vi "COD主界面（列队使用）.vi"() -> (8 "多列列表框":i32(listbox))   [LabVIEW 2016, in "斯坦道CODMn.lvlib"]
uses:
  <vilib>/Analysis/6fits.llb/Curve Fitting Criteria.ctl
  <vilib>/Utility/miscctls.llb/LVPointTypeDef.ctl
  <vilib>/Plasmionique/MB Master/MB_Master_Serial/MB_Master_Serial.lvclass
  F:/Program Files/National Instruments/LabVIEW 2016/vi.lib/Plasmionique/MB Master/MB_Master/MB_Master.lvclass
  <vilib>/Utility/config.llb/Read Key (Double).vi
  <vilib>/Utility/config.llb/Read Key (I32).vi
  <vilib>/Utility/config.llb/Read Key (Boolean).vi
  <vilib>/Utility/config.llb/Write Key (I32).vi
  <vilib>/Utility/config.llb/Write Key (Double).vi
  <vilib>/Utility/config.llb/Write Key (Boolean).vi
  <vilib>/Plasmionique/MB Master/MB Master.lvlib
  <vilib>/ptbypt/NI_PtbyPt.lvlib
  PLC/PLC.lvlib
  <vilib>/Utility/config.llb/NI_LVConfig.lvlib
  <vilib>/Analysis/NI_AALPro.lvlib
panel:
  in  "方程参数写入":bool
  in  "读取方程系数":T1
  out "高量程拟合方程":string
  out "低量程拟合方程":string
  out "测量模式数字":i32
  out "零点核查标记":bool
  out "排液故障":bool
  out "进水样超量程":bool
  out "标样核查标记":bool
  out "平行样测量":bool
  out "加标回收测量":bool
  out "质控样测量":bool
  out "待机":bool
  out "校标错误":bool
  out "校零错误":bool
  out "测量错误":bool
  out "草酸钠报警":bool
  out "高锰酸钾报警":bool
  out "加热故障":bool
  out "温控器故障":bool
  out "ORP故障":bool
  out "排液标记":bool
  out "故障标记":bool
  out "校标标记":bool
  out "校零标记":bool
  out "通讯状态":bool
  out "水样测量":bool
  out "读取KB值":bool
  in  "读取":bool
  out "b 2":dbl
  out "K 2":dbl
  out "b":dbl
  out "K":dbl
  out "当前选用的校准":i32
  in  "启用3":bool
  in  "启用2":bool
  in  "启用1":bool
  in  "启用6":bool
  in  "启用5":bool
  in  "校准6":bool
  in  "校准5":bool
  in  "校准4":bool
  in  "启用4":bool
  in  "泵滴定数6":dbl
  in  "泵滴定数5":dbl
  in  "泵滴定数4":dbl
  in  "浓度6":dbl
  in  "浓度5":dbl
  in  "浓度4":dbl
  in  "校准3":bool
  in  "校准2":bool
  in  "校准1":bool
  in  "泵滴定数3":dbl
  in  "泵滴定数2":dbl
  in  "泵滴定数1":dbl
  in  "浓度3":dbl
  in  "浓度2":dbl
  in  "浓度1":dbl
  in  "返回":bool
  in  "校准配置":bool
  in  "修正系数 2":dbl
  in  "浓度 2":dbl
  in  "温度":dbl
  in  "保存":bool
  in  "恒温时间":dbl
  in  "基本量程":enum16{"10mL", "20mL"}(ring)
  in  "水样":dbl
  in  "蒸馏水":dbl
  in  "标液":dbl
  in  "质控样":dbl
  in  "加标回收":dbl
  in  "草酸钠":dbl
  in  "高锰酸钾":dbl
  in  "硫酸":dbl
  in  "关闭":bool
  in  "零点泵计量数 2":dbl
  in  "标度泵计量数 2":dbl
  out "标度滴定值":dbl
  out "零点滴定值":dbl
  out "测量数据区":T2 {"单位" items=["ug/L", "mg/L", "ppm", "mg/m3", "cm", "ppb", "ug/m3", "%", "nmol/mol", "umol/mol", "MPN/L", "MPN/100ml", "ng/m3", "NTU", "无量纲", "ms/cm", "us/cm", "℃", "mV", "万个/L"]}
  out "启动选择 3":u16(ring) items=["水样测试", "标样核查", "零点核查", "加标回收", "平行样", "校零", "校标", ""]
  out "仪器时间":timestamp
  out "秒":u16
  out "分":u16
  out "COD浓度（mg/L)":dbl format="%.2g"
  out "进样管":dbl
  out "高锰酸钾":dbl
  out "草酸钠":dbl
  out "硫酸":dbl
  out "ORP显示":dbl
  out "温度":dbl
  out "加热":bool
  out "搅拌":bool
  out "进硫酸":bool
  out "进加标回收样":bool
  out "进质控样":bool
  out "进标液":bool
  out "进蒸馏水":bool
  out "进水样":bool
  out "进草酸钠":bool
  out "进高锰酸钾":bool
  in  "定时启动":bool
  in  "启动":bool
  in  "故障清除":bool
  in  "参数配置":bool
  in  "停止":bool
  in  "单步启动":bool
  out "设置值":dbl
  out "系统时间":timestamp
  in  "时间校准":bool
  in  "枚举":enum16{"读取数据", "写入数据", "读取写入DATABASE", "读取参数"}(ring)
  in  "data in":T3
  out "数值":i32
  out "报警簇":T4
  out "读取参数":u16[](array[numeric])
  out "循环次数":i32
  out "DATABASE":u16[](array[numeric])
  out "Registers":u16[](array[numeric])
  in  "Slave ID":u8=1
  in  "Serial Config":T5={"baud rate (bps)"=115200, "stop bits"=10, "parity"=0, "flow control"=0, "timeout"=1000, "retries"=1} {"stop bits" items=["1.0"=10, "1.5"=15, "2.0"=20]; "flow control" items=["None", "XON/XOFF", "RTS/CTS", "XON/XOFF & RTS/CTS", "DTR/DSR", "XON/XOFF & DTR/DSR"]; "parity" items=["None", "Odd", "Even", "Mark", "Space"]}
  out "table 输入":string
  out "columns":string[](array[string])
  out "data":T6
  in  "温度 2":dbl
  in  "浓度":dbl
  in  "修正系数":dbl
  in  "标样浓度 2":dbl
  out "模式（受控）":u16
  in  "VISA resource name":refnum<visa-resource-name>="COM3" caption="VISA资源名称"
  # "测量时间："
  # "水样~加标回收"
  # "mV"
  # "℃"
  # "注：遇到加热故障和排液故障时仪器不能正常启动，\n必须排查故障并点击报警清除按钮方可运行。"
  # "mg/L"
  # "基本参数设置"
  # "泵计量参数设置"
  # "校零校标结果"
  # "加热恒温温度（℃）："
  # "水样："
  # "高锰酸钾："
  # "校零结果："
  # "校零滴定值："
  # "恒温时间（分钟）："
  # "蒸馏水："
  # "草酸钠："
  # "校标结果："
  # "标度滴定值："
  # "零点泵计量值："
  # "标准液浓度（mg/L）："
  # "标液："
  # "硫酸："
  # "标样浓度："
  # "标度泵计量值："
  # "修正系数："
  # "质控样："
  # "加标回收样："
  # "基本量程（20mL可选）："
  # "低量程校准"
  # "高量程校准"
  # "泵滴定数"
  # "是否启用"
  # "泵滴定数"
  # "是否启用"
  # "浓度"
  # "浓度"
  # "将方程写入"
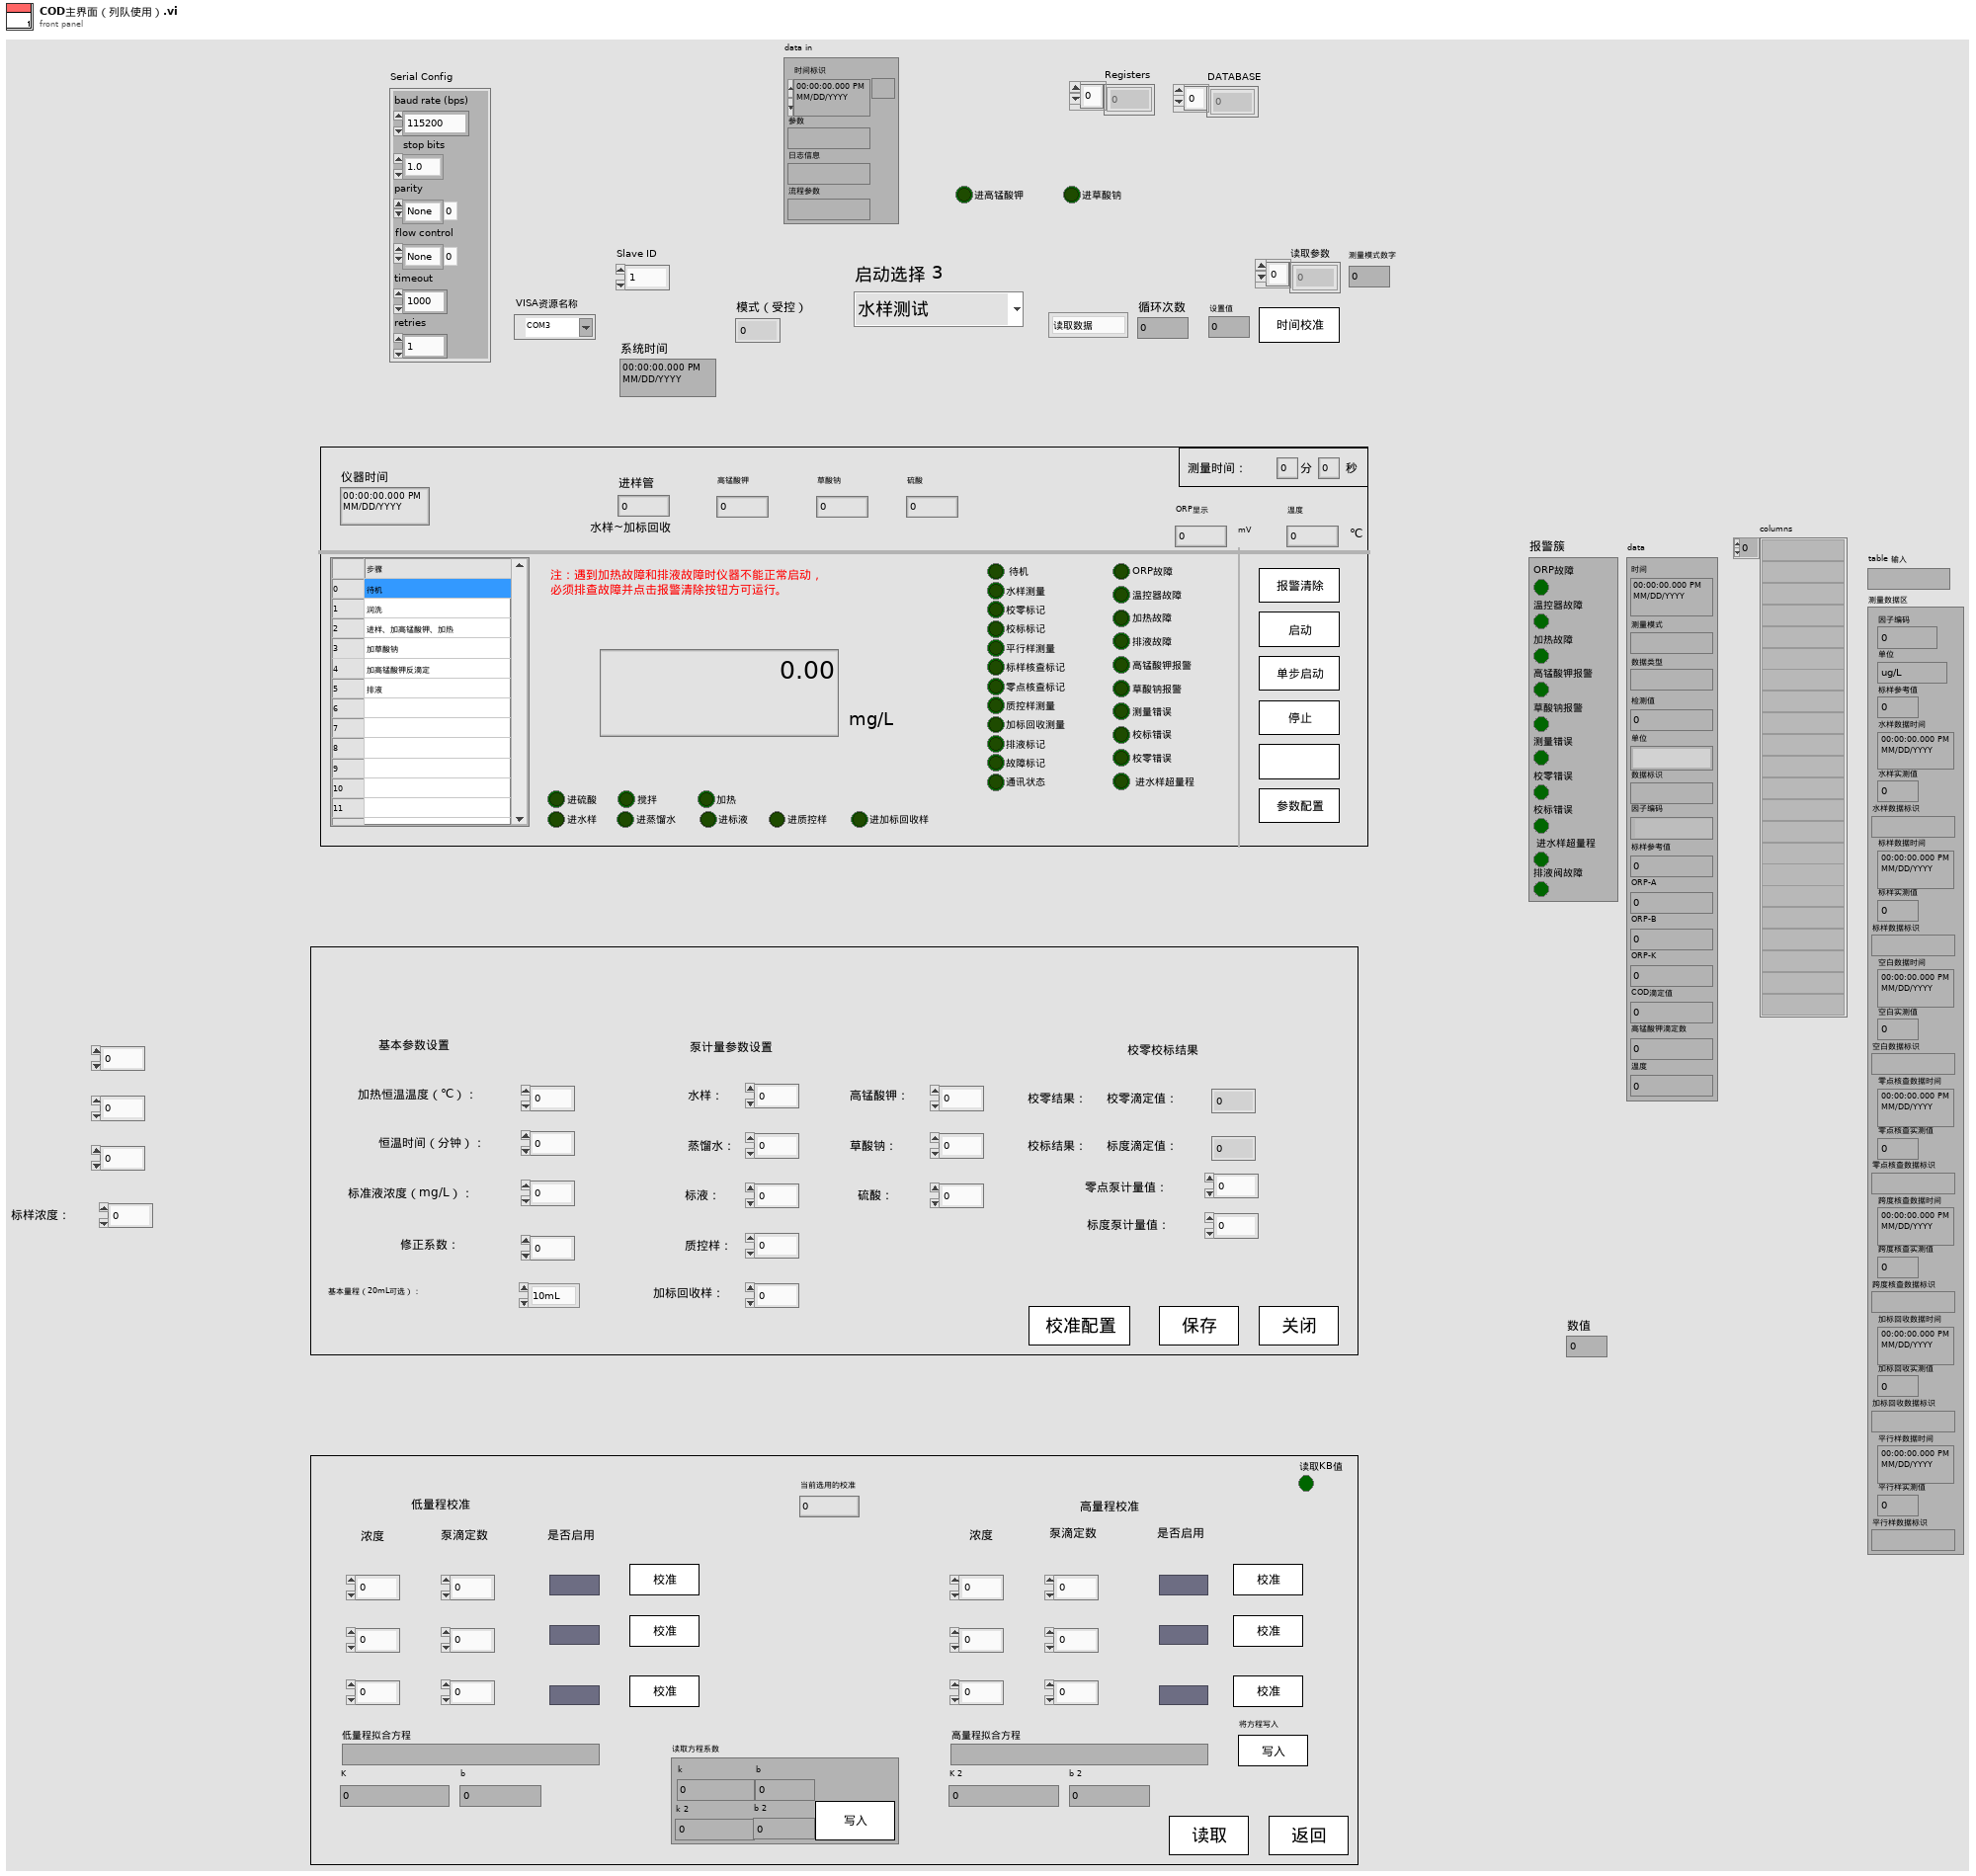
[diagram p1: front panel]
types:
  T1 = cluster{"k":dbl, "b":dbl, "k 2":dbl, "b 2":dbl, "写入":bool}
  T2 = cluster{"因子编码":u32, "单位":u16, "标样参考值":sgl, "水样数据时间":timestamp, "水样实测值":sgl, "水样数据标识":string, "标样数据时间":timestamp, "标样实测值":sgl, "标样数据标识":string, "空白数据时间":timestamp, "空白实测值":sgl, "空白数据标识":string, "零点核查数据时间":timestamp, "零点核查实测值":sgl, "零点核查数据标识":string, "跨度核查数据时间":timestamp, "跨度核查实测值":sgl, "跨度核查数据标识":string, "加标回收数据时间":timestamp, "加标回收实测值":sgl, "加标回收数据标识":string, "平行样数据时间":timestamp, "平行样实测值":sgl, "平行样数据标识":string}
  T3 = cluster{"时间标识":timestamp, "参数":string, "日志信息":string, "流程参数":string}
  T4 = cluster{"ORP故障":bool, "温控器故障":bool, "加热故障":bool, "高锰酸钾报警":bool, "草酸钠报警":bool, "测量错误":bool, "校零错误":bool, "校标错误":bool, " 进水样超量程":bool, "排液阀故障":bool}
  T5 = cluster{"baud rate (bps)":u32, "stop bits":u16, "parity":u16, "flow control":u16, "timeout":u32, "retries":i32}
  T6 = cluster{"时间":timestamp, "测量模式":string, "数据类型":string, "检测值":sgl, "单位":string, "数据标识":string, "因子编码":string, "标样参考值":sgl, "ORP-A":sgl, "ORP-B":sgl, "ORP-K":sgl, "COD滴定值":sgl, "高锰酸钾滴定数":sgl, "温度":sgl}
  T7 = cluster{"starting address":u16, "number of holding registers":u16}
  T8 = typedef "LVPointTypeDef.ctl" = cluster{"Horizontal":i16, "Vertical":i16}
  T9 = cluster{"测量模式":enum16{"水样测量", "标样核查", "零点核查", "加标回收", "平行样", "校零", "校标"}}
  T10 = typedef "NI_LVConfig.lvlib/Config Data RefNum.ctl" = refnum<k1>
  T11 = cluster{"时间标识":timestamp, "设备":string, "日志信息":string}
  T12 = typedef "NI_AALPro.lvlib/Curve Fitting Criteria.ctl" = u16
  T13 = cluster{"时间标识":timestamp, "设备":string, "日志信息":string, "流程参数":string}
  T14 = cluster{"数组 2[0]":sgl, "数组 2[1]":sgl, "数组 2[2]":sgl, "数组 2[3]":sgl}
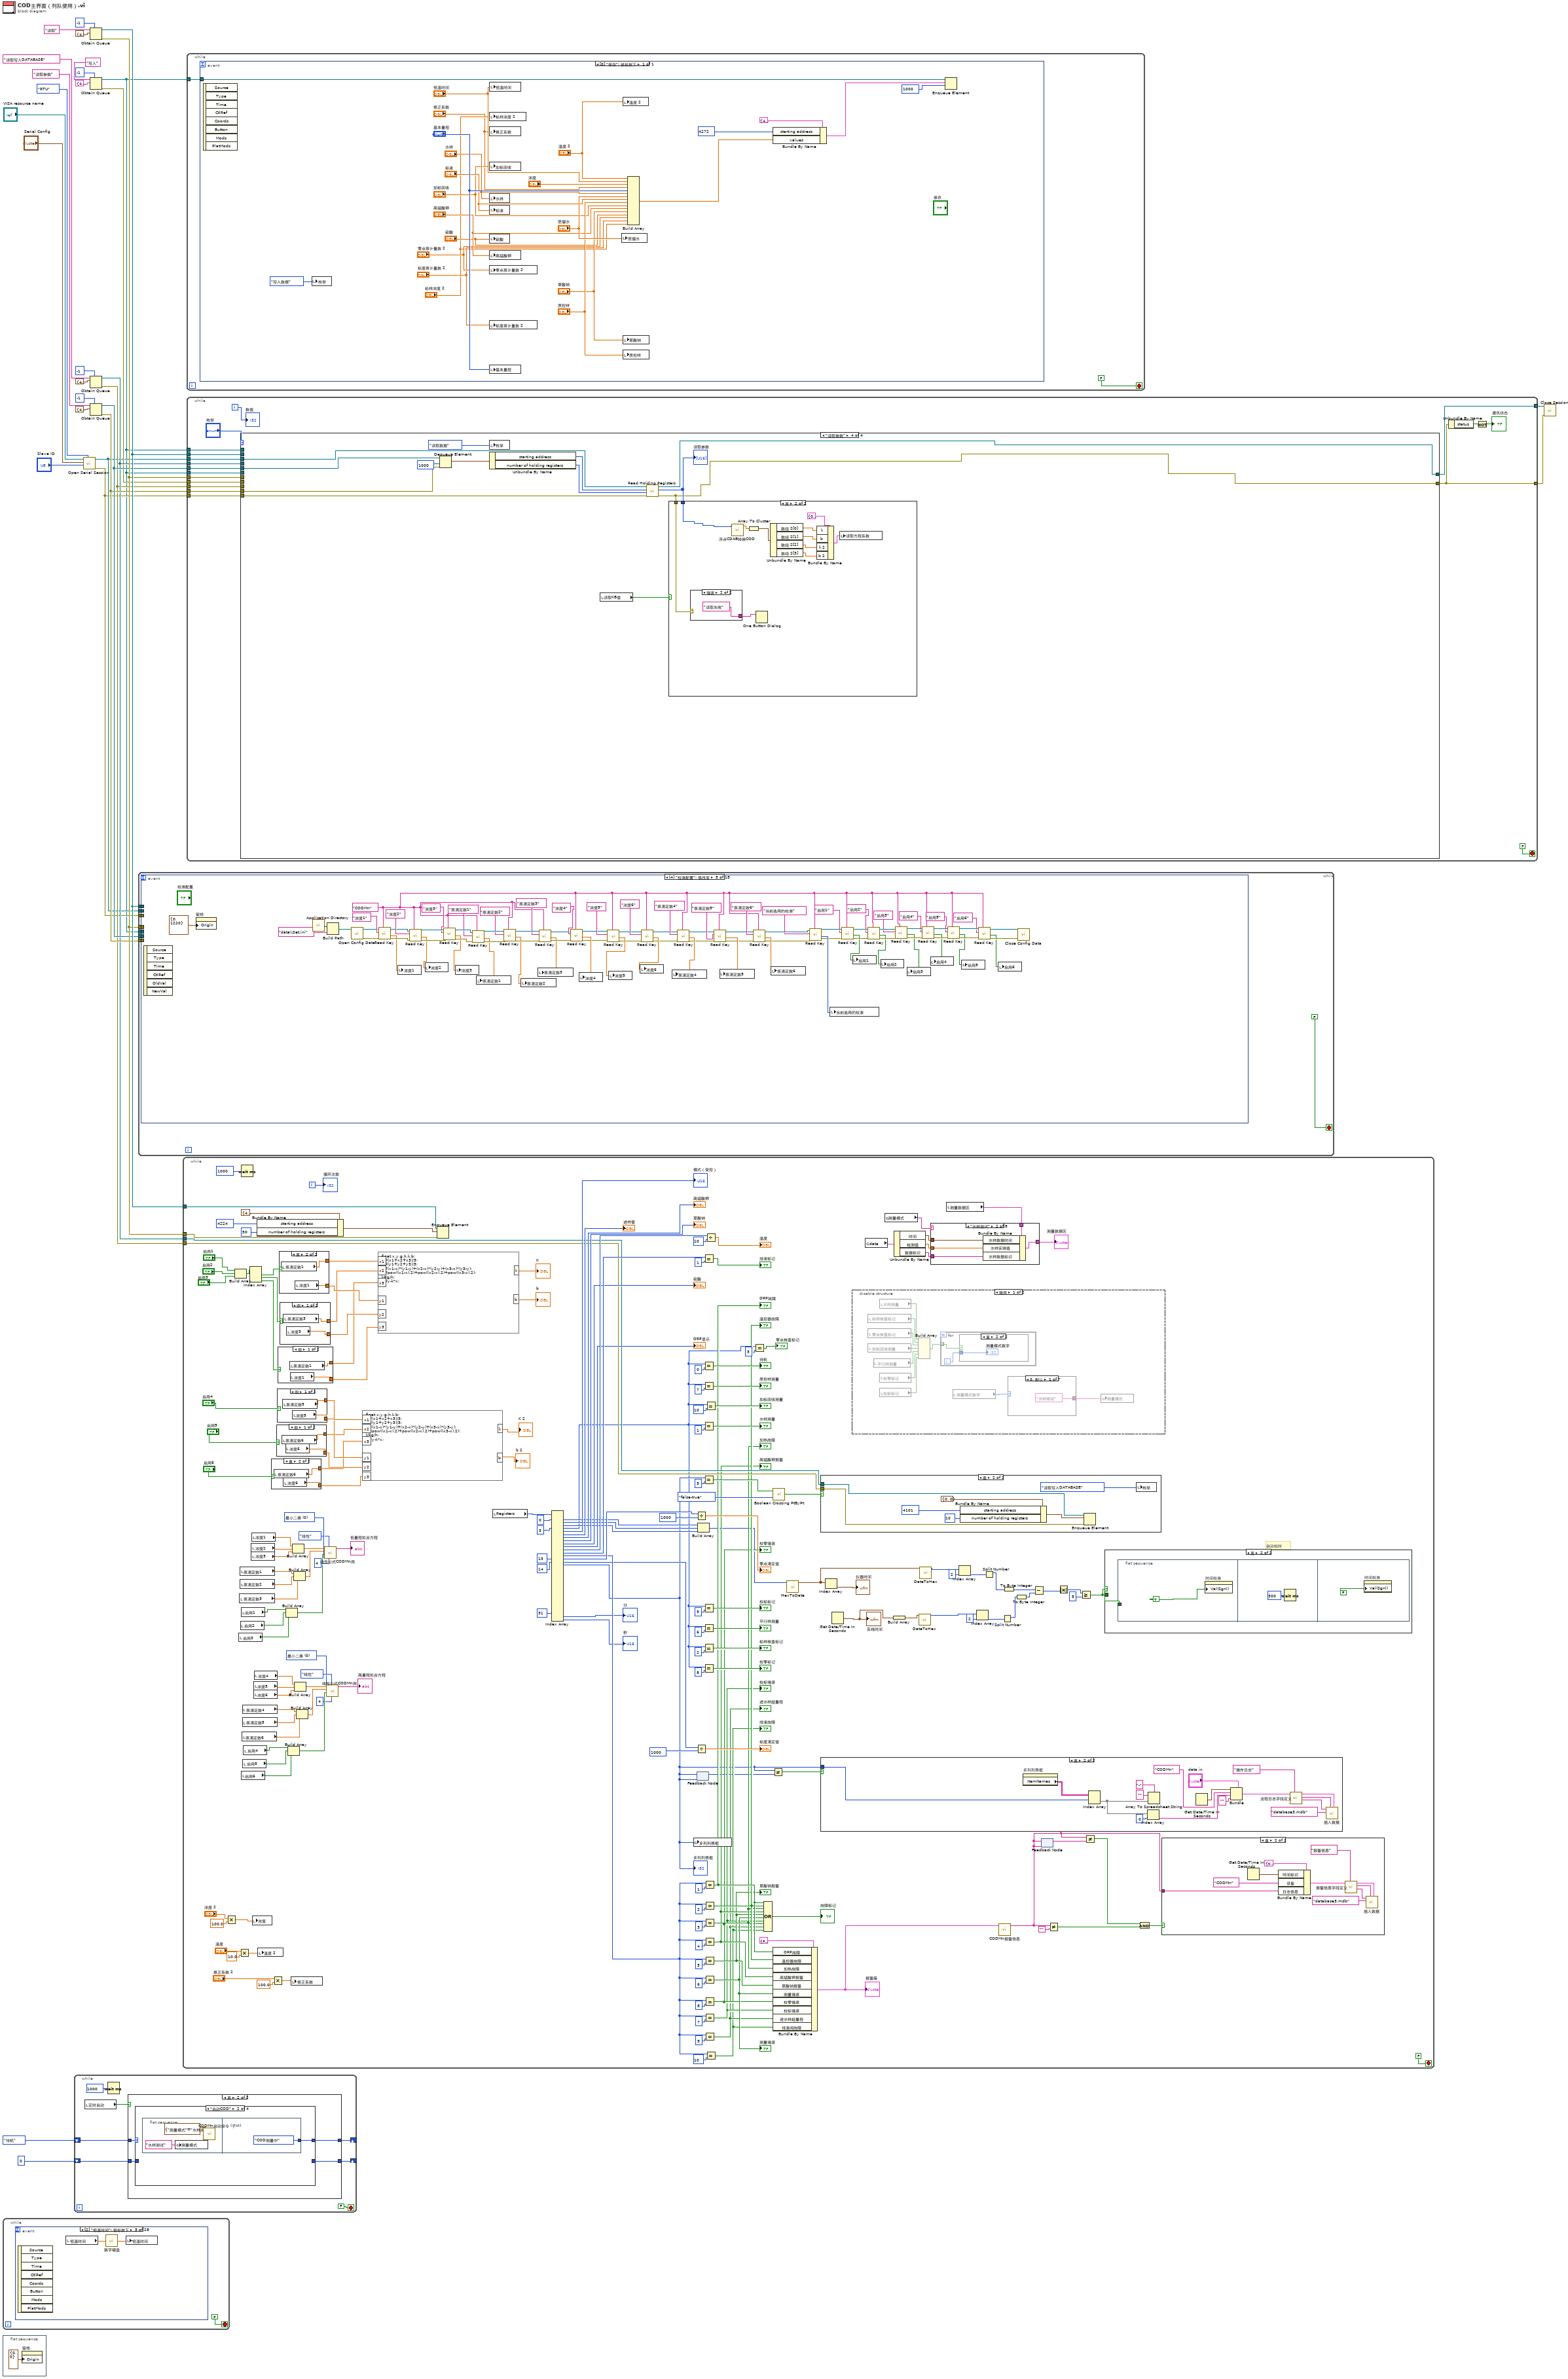
[diagram p0: block diagram]
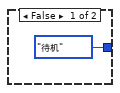
[diagram p2: hidden frame]
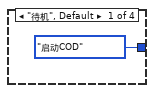
[diagram p3: hidden frame]
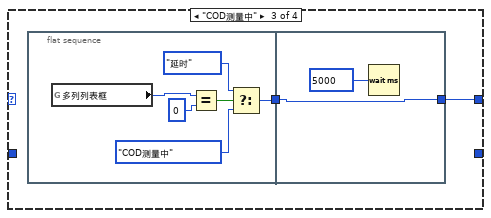
[diagram p4: hidden frame]
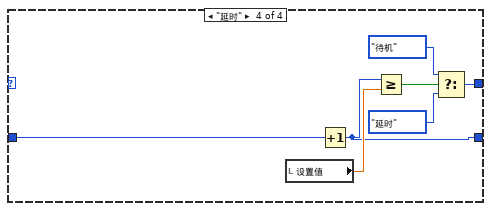
[diagram p5: hidden frame]
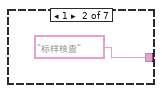
[diagram p6: hidden frame]
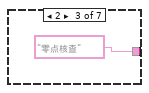
[diagram p7: hidden frame]
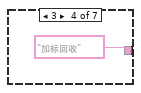
[diagram p8: hidden frame]
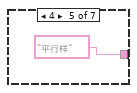
[diagram p9: hidden frame]
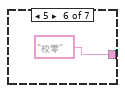
[diagram p10: hidden frame]
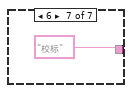
[diagram p11: hidden frame]
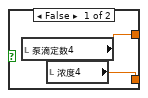
[diagram p14: hidden frame]
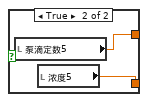
[diagram p15: hidden frame]
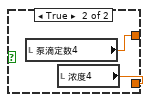
[diagram p16: hidden frame]
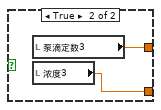
[diagram p17: hidden frame]
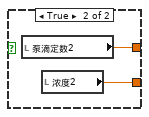
[diagram p18: hidden frame]
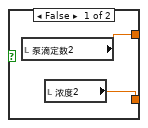
[diagram p19: hidden frame]
diagram:
  n1 = while {
    stop <- FALSE stop-if-true
    n2 = event shown="[2] \"恒温时间\": 鼠标按下" {
      selector: _ -> [_ _ _ _ _ _ _ _ _ _ _ _ _ _ _ _ _ _ _ _ _ _ _ _ _ _ _ _]
      dyn-events: _ -> [_ _ _ _ _ _ _ _ _ _ _ _ _ _ _ _ _ _ _ _ _ _ _ _ _ _ _ _]
      timeout: _ -> [_ _ _ _ _ _ _ _ _ _ _ _ _ _ _ _ _ _ _ _ _ _ _ _ _ _ _ _]
      event Timeout {
        n3 = event-data() -> ()  [unwired: 1 in, 3 out]
      }
      event "温度": Mouse Down {
        n4 = event-data() -> ()  [unwired: 1 in, 8 out]
        n5 = local read "温度"() -> (w33:dbl)
        n6 = call "数字键盘.vi"("OldNumber"=w33) -> ("NewNumber"=w32:sgl)
        n7 = local write "温度"(w32) -> ()
      }
      event "恒温时间": Mouse Down {
        n8 = event-data() -> ()  [unwired: 1 in, 8 out]
        n9 = local read "恒温时间"() -> (w34:dbl)
        n10 = call "数字键盘.vi"("OldNumber"=w34) -> ("NewNumber"=w35:sgl)
        n11 = local write "恒温时间"(w35) -> ()
      }
      event "浓度 2": Mouse Down {
        n12 = event-data() -> ()  [unwired: 1 in, 8 out]
        n13 = local read "浓度 2"() -> (w37:dbl)
        n14 = call "数字键盘.vi"("OldNumber"=w37) -> ("NewNumber"=w36:sgl)
        n15 = local write "浓度 2"(w36) -> ()
      }
      event "修正系数 2": Mouse Down {
        n16 = event-data() -> ()  [unwired: 1 in, 8 out]
        n17 = local read "修正系数 2"() -> (w38:dbl)
        n18 = call "数字键盘.vi"("OldNumber"=w38) -> ("NewNumber"=w39:sgl)
        n19 = local write "修正系数 2"(w39) -> ()
      }
      event "水样": Mouse Down {
        n20 = event-data() -> ()  [unwired: 1 in, 8 out]
        n21 = local read "水样"() -> (w40:dbl)
        n22 = call "数字键盘.vi"("OldNumber"=w40) -> ("NewNumber"=w41:sgl)
        n23 = local write "水样"(w41) -> ()
      }
      event "蒸馏水": Mouse Down {
        n24 = event-data() -> ()  [unwired: 1 in, 8 out]
        n25 = local read "蒸馏水"() -> (w42:dbl)
        n26 = call "数字键盘.vi"("OldNumber"=w42) -> ("NewNumber"=w43:sgl)
        n27 = local write "蒸馏水"(w43) -> ()
      }
      event "标液": Mouse Down {
        n28 = event-data() -> ()  [unwired: 1 in, 8 out]
        n29 = local read "标液"() -> (w44:dbl)
        n30 = call "数字键盘.vi"("OldNumber"=w44) -> ("NewNumber"=w45:sgl)
        n31 = local write "标液"(w45) -> ()
      }
      event "质控样": Mouse Down {
        n32 = event-data() -> ()  [unwired: 1 in, 8 out]
        n33 = local read "质控样"() -> (w46:dbl)
        n34 = call "数字键盘.vi"("OldNumber"=w46) -> ("NewNumber"=w47:sgl)
        n35 = local write "质控样"(w47) -> ()
      }
      event "加标回收": Mouse Down {
        n36 = event-data() -> ()  [unwired: 1 in, 8 out]
        n37 = local read "加标回收"() -> (w48:dbl)
        n38 = call "数字键盘.vi"("OldNumber"=w48) -> ("NewNumber"=w49:sgl)
        n39 = local write "加标回收"(w49) -> ()
      }
      event "草酸钠": Mouse Down {
        n40 = event-data() -> ()  [unwired: 1 in, 8 out]
        n41 = local read "草酸钠"() -> (w50:dbl)
        n42 = call "数字键盘.vi"("OldNumber"=w50) -> ("NewNumber"=w51:sgl)
        n43 = local write "草酸钠"(w51) -> ()
      }
      event "高锰酸钾": Mouse Down {
        n44 = event-data() -> ()  [unwired: 1 in, 8 out]
        n45 = local read "高锰酸钾"() -> (w52:dbl)
        n46 = call "数字键盘.vi"("OldNumber"=w52) -> ("NewNumber"=w53:sgl)
        n47 = local write "高锰酸钾"(w53) -> ()
      }
      event "硫酸": Mouse Down {
        n48 = event-data() -> ()  [unwired: 1 in, 8 out]
        n49 = local read "硫酸"() -> (w54:dbl)
        n50 = call "数字键盘.vi"("OldNumber"=w54) -> ("NewNumber"=w55:sgl)
        n51 = local write "硫酸"(w55) -> ()
      }
      event "零点泵计量数 2": Mouse Down {
        n52 = event-data() -> ()  [unwired: 1 in, 8 out]
        n53 = local read "零点泵计量数 2"() -> (w56:dbl)
        n54 = call "数字键盘.vi"("OldNumber"=w56) -> ("NewNumber"=w57:sgl)
        n55 = local write "零点泵计量数 2"(w57) -> ()
      }
      event "标度泵计量数 2": Mouse Down {
        n56 = event-data() -> ()  [unwired: 1 in, 8 out]
        n57 = local read "标度泵计量数 2"() -> (w58:dbl)
        n58 = call "数字键盘.vi"("OldNumber"=w58) -> ("NewNumber"=w59:sgl)
        n59 = local write "标度泵计量数 2"(w59) -> ()
      }
      event "标样浓度 2": Mouse Down {
        n60 = event-data() -> ()  [unwired: 1 in, 8 out]
        n61 = local read "标样浓度 2"() -> (w60:dbl)
        n62 = call "数字键盘.vi"("OldNumber"=w60) -> ("NewNumber"=w61:sgl)
        n63 = local write "标样浓度 2"(w61) -> ()
      }
      event "浓度1": Mouse Down {
        n64 = event-data() -> ()  [unwired: 1 in, 8 out]
        n65 = local read "浓度1"() -> (w63:dbl)
        n66 = call "数字键盘.vi"("OldNumber"=w63) -> ("NewNumber"=w62:sgl)
        n67 = property on="浓度1" class="DigNum (严格)"("Val(Sgnl)"=w62) -> ()  [unwired: 2 in, 2 out]
      }
      event "浓度2": Mouse Down {
        n68 = event-data() -> ()  [unwired: 1 in, 8 out]
        n69 = local read "浓度2"() -> (w65:dbl)
        n70 = call "数字键盘.vi"("OldNumber"=w65) -> ("NewNumber"=w64:sgl)
        n71 = property on="浓度2" class="DigNum (严格)"("Val(Sgnl)"=w64) -> ()  [unwired: 2 in, 2 out]
      }
      event "浓度3": Mouse Down {
        n72 = event-data() -> ()  [unwired: 1 in, 8 out]
        n73 = local read "浓度3"() -> (w67:dbl)
        n74 = call "数字键盘.vi"("OldNumber"=w67) -> ("NewNumber"=w66:sgl)
        n75 = property on="浓度3" class="DigNum (严格)"("Val(Sgnl)"=w66) -> ()  [unwired: 2 in, 2 out]
      }
      event "泵滴定数1": Mouse Down {
        n76 = event-data() -> ()  [unwired: 1 in, 8 out]
        n77 = local read "泵滴定数1"() -> (w69:dbl)
        n78 = call "数字键盘.vi"("OldNumber"=w69) -> ("NewNumber"=w68:sgl)
        n79 = property on="泵滴定数1" class="DigNum (严格)"("Val(Sgnl)"=w68) -> ()  [unwired: 2 in, 2 out]
      }
      event "泵滴定数2": Mouse Down {
        n80 = event-data() -> ()  [unwired: 1 in, 8 out]
        n81 = local read "泵滴定数2"() -> (w71:dbl)
        n82 = call "数字键盘.vi"("OldNumber"=w71) -> ("NewNumber"=w70:sgl)
        n83 = property on="泵滴定数2" class="DigNum (严格)"("Val(Sgnl)"=w70) -> ()  [unwired: 2 in, 2 out]
      }
      event "泵滴定数3": Mouse Down {
        n84 = event-data() -> ()  [unwired: 1 in, 8 out]
        n85 = local read "泵滴定数3"() -> (w73:dbl)
        n86 = call "数字键盘.vi"("OldNumber"=w73) -> ("NewNumber"=w72:sgl)
        n87 = property on="泵滴定数3" class="DigNum (严格)"("Val(Sgnl)"=w72) -> ()  [unwired: 2 in, 2 out]
      }
      event "浓度4": Mouse Down {
        n88 = event-data() -> ()  [unwired: 1 in, 8 out]
        n89 = local read "浓度4"() -> (w75:dbl)
        n90 = call "数字键盘.vi"("OldNumber"=w75) -> ("NewNumber"=w74:sgl)
        n91 = property on="浓度4" class="DigNum (严格)"("Val(Sgnl)"=w74) -> ()  [unwired: 2 in, 2 out]
      }
      event "浓度5": Mouse Down {
        n92 = event-data() -> ()  [unwired: 1 in, 8 out]
        n93 = local read "浓度5"() -> (w77:dbl)
        n94 = call "数字键盘.vi"("OldNumber"=w77) -> ("NewNumber"=w76:sgl)
        n95 = property on="浓度5" class="DigNum (严格)"("Val(Sgnl)"=w76) -> ()  [unwired: 2 in, 2 out]
      }
      event "浓度6": Mouse Down {
        n96 = event-data() -> ()  [unwired: 1 in, 8 out]
        n97 = local read "浓度6"() -> (w79:dbl)
        n98 = call "数字键盘.vi"("OldNumber"=w79) -> ("NewNumber"=w78:sgl)
        n99 = property on="浓度6" class="DigNum (严格)"("Val(Sgnl)"=w78) -> ()  [unwired: 2 in, 2 out]
      }
      event "泵滴定数4": Mouse Down {
        n100 = event-data() -> ()  [unwired: 1 in, 8 out]
        n101 = local read "泵滴定数4"() -> (w81:dbl)
        n102 = call "数字键盘.vi"("OldNumber"=w81) -> ("NewNumber"=w80:sgl)
        n103 = property on="泵滴定数4" class="DigNum (严格)"("Val(Sgnl)"=w80) -> ()  [unwired: 2 in, 2 out]
      }
      event "泵滴定数5": Mouse Down {
        n104 = event-data() -> ()  [unwired: 1 in, 8 out]
        n105 = local read "泵滴定数5"() -> (w83:dbl)
        n106 = call "数字键盘.vi"("OldNumber"=w83) -> ("NewNumber"=w82:sgl)
        n107 = property on="泵滴定数5" class="DigNum (严格)"("Val(Sgnl)"=w82) -> ()  [unwired: 2 in, 2 out]
      }
      event "泵滴定数6": Mouse Down {
        n108 = event-data() -> ()  [unwired: 1 in, 8 out]
        n109 = local read "泵滴定数6"() -> (w85:dbl)
        n110 = call "数字键盘.vi"("OldNumber"=w85) -> ("NewNumber"=w84:sgl)
        n111 = property on="泵滴定数6" class="DigNum (严格)"("Val(Sgnl)"=w84) -> ()  [unwired: 2 in, 2 out]
      }
    }
  }
  n112 = flat-sequence {
    frame #0 {
      n113 = property on="窗格" class="Pane"("Origin"=T8 {"Horizontal"=0, "Vertical"=0} ("原点")) -> ()  [unwired: 2 in, 2 out]
    }
  }
  n114 = while {
    shift-right: [w88] -> _
    shift-left: enum16{"待机", "启动COD", "COD测量中", "延时"}."待机" -> [w90]
    shift-right: [w87] -> _
    shift-left: 0 -> [w89]
    stop <- FALSE stop-if-true
    n115 = local read "定时启动"() -> (w92:bool)
    n116 = Wait (ms)(milliseconds to wait=u32 1000 ("等待时间（毫秒）")) -> ()  [unwired: 1 out]
    n117 = case shown="真" w92 {
      tunnel: w90 -> [_ w98]
      tunnel: w89 -> [_ w97]
      tunnel: [enum16{"待机", "启动COD", "COD测量中", "延时"}."待机" w96] -> w88
      tunnel: [_ w95] -> w87
      frame False {
      }
      frame True {
        n118 = case shown="\"启动COD\"" w98 {
          tunnel: w97 -> [_ _ _ w120]
          tunnel: [enum16{"待机", "启动COD", "COD测量中", "延时"}."启动COD" w100 w105 w114] -> w96
          tunnel: [_ _ _ w117] -> w95
          frame "待机", Default {
          }
          frame "启动COD" {
            n119 = flat-sequence {
              tunnel: [enum16{"待机", "启动COD", "COD测量中", "延时"}."COD测量中"] -> w100
              frame #0 {
                n120 = global write "COD测量模式全局.vi" "测量模式"("水样测试" ("测量模式")) -> ()
                n121 = call "CODMn启动命令 (子VI).vi"("启动测量模式"=T9 {"测量模式"=enum."水样测量"}) -> ()  [unwired: 11 in]
              }
              frame #1 {
              }
            }
          }
          frame "COD测量中" {
            n122 = flat-sequence {
              tunnel: [w106] -> w104
              tunnel: [w113] -> w105
              tunnel: w104 -> [w113]
              frame #0 {
                n123 = global read "运行时序全局变量.vi" "多列列表框"() -> (w111:i32)
                n124 = Equal?(x=w111, y=0) -> (x = y?=w109:bool)
                n125 = Select(t=enum16{"待机", "启动COD", "COD测量中", "延时"}."延时", s=w109, f=enum16{"待机", "启动COD", "COD测量中", "延时"}."COD测量中") -> (s? t:f=w106:enum16{"待机", "启动COD", "COD测量中", "延时"})
              }
              frame #1 {
                n126 = Wait (ms)(milliseconds to wait=u32 5000 ("等待时间（毫秒）")) -> ()  [unwired: 1 out]
              }
            }
          }
          frame "延时" {
            n127 = local read "设置值"() -> (w119:dbl)
            n128 = Increment(x=w120) -> (x+1=w117:i32)
            n129 = Greater Or Equal?(x=w117, y=w119) -> (x >= y?=w118:bool)
            n130 = Select(t=enum16{"待机", "启动COD", "COD测量中", "延时"}."待机", s=w118, f=enum16{"待机", "启动COD", "COD测量中", "延时"}."延时") -> (s? t:f=w114:enum16{"待机", "启动COD", "COD测量中", "延时"})
          }
        }
      }
    }
  }
  n131 = call <vilib>:"Open Serial Session.vi"("Mode (RTU)"=enum16{"RTU", "ASCII"}."RTU", "Slave ID"="Slave ID", "Serial Config"="Serial Config", "VISA Resource"="VISA resource name") -> ("Error out"=w4:errorcluster, "MB_Serial session"=w5:refnum<class "MB_Master_Serial.lvclass">)  [unwired: 6 in]
  n132 = Obtain Queue(max queue size (-1, unlimited)=-1 ("队列最大值（-1，无限）"), name (unnamed)="读取" ("名称（未命名）"), element data type=T7 {"starting address"=4224, "number of holding registers"=16}) -> (queue out=w20:refnum<queue>, error out=w19:errorcluster)  [unwired: 2 in, 1 out]
  n133 = Obtain Queue(max queue size (-1, unlimited)=-1 ("队列最大值（-1，无限）"), name (unnamed)="写入" ("名称（未命名）"), element data type=cluster{"starting address":u16, "values":u16[]} {"starting address"=4272, "values"=[]}) -> (queue out=w1:refnum<queue>, error out=w6:errorcluster)  [unwired: 2 in, 1 out]
  n134 = Obtain Queue(max queue size (-1, unlimited)=-1 ("队列最大值（-1，无限）"), name (unnamed)="读取写入DATABASE" ("名称（未命名）"), element data type=T7 {"starting address"=4224, "number of holding registers"=16}) -> (queue out=w8:refnum<queue>, error out=w7:errorcluster)  [unwired: 2 in, 1 out]
  n135 = Obtain Queue(max queue size (-1, unlimited)=-1 ("队列最大值（-1，无限）"), name (unnamed)="读取参数" ("名称（未命名）"), element data type=T7 {"starting address"=4224, "number of holding registers"=16}) -> (queue out=w13:refnum<queue>, error out=w12:errorcluster)  [unwired: 2 in, 1 out]
  n136 = while {
    tunnel: w20 -> [w128]
    tunnel: w19 -> [w127]
    tunnel: w1 -> [w126]
    tunnel: w13 -> [w125]
    tunnel: w12 -> [w124]
    tunnel: w5 -> [w122]
    tunnel: w4 -> [w121]
    stop <- FALSE stop-if-true
    n137 = event shown="[4] \"校准配置\": 值改变" {
      selector: _ -> [_ _ _ _ _ _ _ _ _ _ _ _ _ _ _]
      dyn-events: _ -> [_ _ _ _ _ _ _ _ _ _ _ _ _ _ _]
      timeout: _ -> [_ _ _ _ _ _ _ _ _ _ _ _ _ _ _]
      tunnel: w128 -> [_ _ _ _ _ _ _ _ _ _ _ _ _ _ _]
      tunnel: w127 -> [_ _ _ _ _ _ _ _ _ _ _ _ _ _ _]
      tunnel: w126 -> [w135 w163 w194 _ _ _ _ w297 w311 _ w319 _ _ w479 w496]
      tunnel: w125 -> [_ _ _ w201 _ _ _ _ _ _ _ _ w471 _ _]
      tunnel: w124 -> [_ _ _ w200 _ _ _ _ _ _ _ _ w470 _ _]
      tunnel: w122 -> [_ _ _ _ _ _ w296 _ _ _ _ _ _ _ _]
      tunnel: w121 -> [_ _ _ _ _ _ w295 _ _ _ _ _ _ _ _]
      event "单步启动": Mouse Down {
        n138 = event-data() -> ()  [unwired: 1 in, 8 out]
        n139 = call "单步启动选择对话框.vi"() -> ("启动选择 2"=w138:u16)  [unwired: 10 in, 1 out]
        n140 = case shown="0" w138 {
          tunnel: [u16 4610 ("address") u16 4610 ("address") u16 4610 ("address") u16 4610 ("address") u16 4610 ("address") u16 4610 ("address") u16 4610 ("address") u16 4610 ("address") u16 4610 ("address") u16 4610 ("address") u16 4610 ("address") u16 4610 ("address")] -> w134
          tunnel: [u16 1 ("address") u16 2 ("address") u16 3 ("address") u16 4 ("address") u16 5 ("address") u16 6 ("address") u16 7 ("address") u16 8 ("address") u16 9 ("holding register value") u16 10 ("holding register value") u16 11 ("holding register value") u16 0 ("address")] -> w131
          frame 0 {
          }
          frame 1 {
          }
          frame 2 {
          }
          frame 3 {
          }
          frame 4 {
          }
          frame 5 {
          }
          frame 6 {
          }
          frame 7 {
          }
          frame 8 {
          }
          frame 9 {
          }
          frame 10 {
          }
          frame 11, Default {
          }
        }
        n141 = local write "枚举"(enum16{"读取数据", "写入数据", "读取写入DATABASE", "读取参数"}."写入数据" ("枚举")) -> ()
        n142 = Insert Into Array(array=u16[] [] ("values"), index=0 ("索引"), new element=w131) -> (w130:u16[])
        n143 = Bundle By Name(cluster=cluster{"starting address":u16, "values":u16[]} {"starting address"=0, "values"=[]}, "starting address"=w134, "values"=w130) -> (w136:cluster{"starting address":u16, "values":u16[]})
        n144 = Enqueue Element(queue=w135, element=w136) -> ()  [unwired: 2 in, 3 out]
      }
      event "启动": Mouse Down {
        n145 = event-data() -> ()  [unwired: 1 in, 8 out]
        n146 = flat-sequence {
          tunnel: [w166] -> w164
          tunnel: w164 -> [w175]
          tunnel: w163 -> [w169]
          frame #0 {
            n147 = call "启动测量模式选择对话框.vi"() -> ("启动选择 3"=w166:u16)  [unwired: 11 in]
            "启动选择 3" <- w166
          }
          frame #1 {
            n148 = property on="启动选择 3" class="Ring (严格)"() -> ("RingText.Text"=w176:string)  [unwired: 2 in, 2 out]
            n149 = case shown="6" w175 {
              tunnel: [u16 4608 ("address") u16 4608 ("address") u16 4608 ("address") u16 4608 ("address") u16 4608 ("address") u16 4608 ("address") u16 4608 ("address") u16 4608 ("address")] -> w167
              tunnel: [u16 1 ("address") u16 2 ("address") u16 3 ("address") u16 7 ("address") u16 6 ("address") u16 8 ("address") u16 9 ("address") u16 0 ("address")] -> w168
              frame 0 {
              }
              frame 1 {
              }
              frame 2 {
              }
              frame 3 {
              }
              frame 4 {
              }
              frame 5 {
              }
              frame 6 {
              }
              frame 7, Default {
              }
            }
            n150 = global write "COD测量模式全局.vi" "测量模式"(w176) -> ()
            n151 = Insert Into Array(array=u16[] [] ("values"), index=0 ("索引"), new element=w168) -> (w174:u16[])
            n152 = Bundle By Name(cluster=cluster{"starting address":u16, "values":u16[]} {"starting address"=0, "values"=[]}, "starting address"=w167, "values"=w174) -> (w171:cluster{"starting address":u16, "values":u16[]})
            n153 = Enqueue Element(queue=w169, element=w171) -> ()  [unwired: 2 in, 3 out]
          }
        }
        n154 = local write "枚举"(enum16{"读取数据", "写入数据", "读取写入DATABASE", "读取参数"}."写入数据" ("枚举")) -> ()
      }
      event "停止": Value Change {
        n155 = event-data() -> ()  [unwired: 1 in, 6 out]
        n156 = local write "枚举"(enum16{"读取数据", "写入数据", "读取写入DATABASE", "读取参数"}."写入数据" ("枚举")) -> ()
        n157 = Bundle By Name(cluster=cluster{"starting address":u16, "values":u16[]} {"starting address"=0, "values"=[]}, "starting address"=u16 4608, "values"=u16[] [11]) -> (w196:cluster{"starting address":u16, "values":u16[]})
        n158 = Enqueue Element(queue=w194, element=w196) -> ()  [unwired: 2 in, 3 out]
      }
      event "参数配置": Value Change {
        n159 = event-data() -> ()  [unwired: 1 in, 6 out]
        n160 = property on="窗格" class="Pane"("Origin"=T8 {"Horizontal"=0, "Vertical"=610} ("原点")) -> ()  [unwired: 2 in, 2 out]
        n161 = Bundle By Name(cluster=T7 {"starting address"=0, "number of holding registers"=0}, "starting address"=u16 4240, "number of holding registers"=u16 16) -> (w208:T7)
        n162 = local write "枚举"(enum16{"读取数据", "写入数据", "读取写入DATABASE", "读取参数"}."读取参数" ("枚举")) -> ()
        n163 = Flush Queue(queue=w201, error in (no error)=w200) -> (queue out=w204:refnum<queue>, error out=w203:errorcluster)  [unwired: 1 out]
        n164 = Enqueue Element(queue=w204, element=w208, error in (no error)=w203) -> ()  [unwired: 1 in, 3 out]
        n165 = local write "读取KB值"(FALSE ("读取KB值")) -> ()
      }
      event "校准配置": Value Change {
        w223 = "CODMn" ("section")
        n166 = event-data() -> ()  [unwired: 1 in, 6 out]
        n167 = property on="窗格" class="Pane"("Origin"=T8 {"Horizontal"=0, "Vertical"=1220} ("原点")) -> ()  [unwired: 2 in, 2 out]
        n168 = call <vilib>:"Application Directory.vi"() -> ("Application Directory"=w243:path)
        n169 = Build Path(base path=w243, name or relative path="data\\Set.ini" ("名称或相对路径")) -> (appended path=w241:path)
        n170 = call <vilib>:"Open Config Data.vi"("configuration file path"=w241) -> ("error out"=w244:errorcluster, "refnum"=w245:T10)  [unwired: 8 in, 1 out]
        n171 = call-poly <vilib>:"Read Key.vi"("section"=w223, "error in (no error)"=w244, "key"="浓度1", "refnum"=w245) -> ("error out"=w249:errorcluster, "value"=w247:dbl, "refnum out"=w248:T10)  [unwired: 4 in, 1 out]
        n172 = local write "浓度1"(w247) -> ()
        n173 = call-poly <vilib>:"Read Key.vi"("section"=w223, "error in (no error)"=w249, "key"="浓度2", "refnum"=w248) -> ("error out"=w263:errorcluster, "value"=w250:dbl, "refnum out"=w262:T10)  [unwired: 4 in, 1 out]
        n174 = local write "浓度2"(w250) -> ()
        n175 = call-poly <vilib>:"Read Key.vi"("section"=w223, "error in (no error)"=w263, "key"="浓度3", "refnum"=w262) -> ("error out"=w264:errorcluster, "value"=w252:dbl, "refnum out"=w261:T10)  [unwired: 4 in, 1 out]
        n176 = local write "浓度3"(w252) -> ()
        n177 = call-poly <vilib>:"Read Key.vi"("section"=w223, "error in (no error)"=w264, "key"="泵滴定数1", "refnum"=w261) -> ("error out"=w265:errorcluster, "value"=w254:dbl, "refnum out"=w260:T10)  [unwired: 4 in, 1 out]
        n178 = local write "泵滴定数1"(w254) -> ()
        n179 = call-poly <vilib>:"Read Key.vi"("section"=w223, "error in (no error)"=w265, "key"="泵滴定数2", "refnum"=w260) -> ("error out"=w259:errorcluster, "value"=w257:dbl, "refnum out"=w266:T10)  [unwired: 4 in, 1 out]
        n180 = local write "泵滴定数2"(w257) -> ()
        n181 = call-poly <vilib>:"Read Key.vi"("section"=w223, "error in (no error)"=w259, "key"="泵滴定数3", "refnum"=w266) -> ("error out"=w274:errorcluster, "value"=w273:dbl, "refnum out"=w267:T10)  [unwired: 4 in, 1 out]
        n182 = local write "泵滴定数3"(w273) -> ()
        n183 = call-poly <vilib>:"Read Key.vi"("section"=w223, "error in (no error)"=w274, "key"="浓度4", "refnum"=w267) -> ("error out"=w275:errorcluster, "value"=w281:dbl, "refnum out"=w268:T10)  [unwired: 4 in, 1 out]
        n184 = local write "浓度4"(w281) -> ()
        n185 = call-poly <vilib>:"Read Key.vi"("section"=w223, "error in (no error)"=w275, "key"="浓度5", "refnum"=w268) -> ("error out"=w276:errorcluster, "value"=w282:dbl, "refnum out"=w269:T10)  [unwired: 4 in, 1 out]
        n186 = local write "浓度5"(w282) -> ()
        n187 = call-poly <vilib>:"Read Key.vi"("section"=w223, "error in (no error)"=w276, "key"="浓度6", "refnum"=w269) -> ("error out"=w277:errorcluster, "value"=w283:dbl, "refnum out"=w270:T10)  [unwired: 4 in, 1 out]
        n188 = local write "浓度6"(w283) -> ()
        n189 = call-poly <vilib>:"Read Key.vi"("section"=w223, "error in (no error)"=w277, "key"="泵滴定数4", "refnum"=w270) -> ("error out"=w278:errorcluster, "value"=w284:dbl, "refnum out"=w271:T10)  [unwired: 4 in, 1 out]
        n190 = local write "泵滴定数4"(w284) -> ()
        n191 = call-poly <vilib>:"Read Key.vi"("section"=w223, "error in (no error)"=w278, "key"="泵滴定数5", "refnum"=w271) -> ("error out"=w279:errorcluster, "value"=w285:dbl, "refnum out"=w272:T10)  [unwired: 4 in, 1 out]
        n192 = local write "泵滴定数5"(w285) -> ()
        n193 = call-poly <vilib>:"Read Key.vi"("section"=w223, "error in (no error)"=w279, "key"="泵滴定数6", "refnum"=w272) -> ("error out"=w237:errorcluster, "value"=w286:dbl, "refnum out"=w240:T10)  [unwired: 4 in, 1 out]
        n194 = local write "泵滴定数6"(w286) -> ()
        n195 = call-poly <vilib>:"Read Key.vi"("section"=w223, "error in (no error)"=w237, "key"="当前选用的校准", "refnum"=w240) -> ("error out"=w235:errorcluster, "value"=w238:i32, "refnum out"=w236:T10)  [unwired: 4 in, 1 out]
        n196 = local write "当前选用的校准"(w238) -> ()
        n197 = call-poly <vilib>:"Read Key.vi"("section"=w223, "error in (no error)"=w235, "key"="启用1", "refnum"=w236) -> ("error out"=w232:errorcluster, "value"=w215:bool, "refnum out"=w233:T10)  [unwired: 4 in, 1 out]
        n198 = local write "启用1"(w215) -> ()
        n199 = call-poly <vilib>:"Read Key.vi"("section"=w223, "error in (no error)"=w232, "key"="启用2", "refnum"=w233) -> ("error out"=w230:errorcluster, "value"=w214:bool, "refnum out"=w231:T10)  [unwired: 4 in, 1 out]
        n200 = local write "启用2"(w214) -> ()
        n201 = call-poly <vilib>:"Read Key.vi"("section"=w223, "error in (no error)"=w230, "key"="启用3", "refnum"=w231) -> ("error out"=w228:errorcluster, "value"=w213:bool, "refnum out"=w229:T10)  [unwired: 4 in, 1 out]
        n202 = local write "启用3"(w213) -> ()
        n203 = call-poly <vilib>:"Read Key.vi"("section"=w223, "error in (no error)"=w228, "key"="启用4", "refnum"=w229) -> ("error out"=w226:errorcluster, "value"=w212:bool, "refnum out"=w227:T10)  [unwired: 4 in, 1 out]
        n204 = local write "启用4"(w212) -> ()
        n205 = call-poly <vilib>:"Read Key.vi"("section"=w223, "error in (no error)"=w226, "key"="启用5", "refnum"=w227) -> ("error out"=w224:errorcluster, "value"=w211:bool, "refnum out"=w225:T10)  [unwired: 4 in, 1 out]
        n206 = local write "启用5"(w211) -> ()
        n207 = call-poly <vilib>:"Read Key.vi"("section"=w223, "error in (no error)"=w224, "key"="启用6", "refnum"=w225) -> ("error out"=w216:errorcluster, "value"=w210:bool, "refnum out"=w217:T10)  [unwired: 4 in, 1 out]
        n208 = local write "启用6"(w210) -> ()
        n209 = call <vilib>:"Close Config Data.vi"("error in (no error)"=w216, "refnum"=w217) -> ()  [unwired: 8 in, 2 out]
      }
      event "返回", "关闭": Value Change {
        n210 = event-data() -> ()  [unwired: 1 in, 6 out]
        n211 = property on="窗格" class="Pane"("Origin"=T8 {"Horizontal"=0, "Vertical"=0} ("原点")) -> ()  [unwired: 2 in, 2 out]
        n212 = local write "读取KB值"(FALSE ("读取KB值")) -> ()
      }
      event Timeout; Application Instance Close {
        n213 = event-data() -> ()  [unwired: 1 in, 3 out]
        n214 = call-dynamic "Close Session.vi"("error in (no error)"=w295, "MB_Serial session"=w296) -> ()  [unwired: 9 in, 1 out]
      }
      event "时间校准": Value Change {
        n215 = event-data() -> ()  [unwired: 1 in, 6 out]
        n216 = flat-sequence {
          tunnel: w297 -> [w302]
          frame #0 {
            n217 = Get Date/Time In Seconds() -> (seconds since 1Jan1904=w307:timestamp)
            n218 = Build Array(w307) -> (w306:timestamp[])
            n219 = call "DateToHex.vi"("DATE"=w306) -> ("数组"=w300:u16[])  [unwired: 10 in]
            n220 = Insert Into Array(array=u16[] [1] ("values"), index=1 ("索引"), new element=w300) -> (w298:u16[])
            n221 = Bundle By Name(cluster=cluster{"starting address":u16, "values":u16[]} {"starting address"=0, "values"=[]}, "starting address"=u16 4612, "values"=w298) -> (w303:cluster{"starting address":u16, "values":u16[]})
            n222 = Enqueue Element(queue=w302, element=w303) -> ()  [unwired: 2 in, 3 out]
          }
          frame #1 {
            n223 = local write "枚举"(enum16{"读取数据", "写入数据", "读取写入DATABASE", "读取参数"}."写入数据" ("枚举")) -> ()
          }
        }
      }
      event "故障清除": Value Change {
        n224 = event-data() -> ()  [unwired: 1 in, 6 out]
        n225 = local write "枚举"(enum16{"读取数据", "写入数据", "读取写入DATABASE", "读取参数"}."写入数据" ("枚举")) -> ()
        n226 = Bundle By Name(cluster=cluster{"starting address":u16, "values":u16[]} {"starting address"=0, "values"=[]}, "starting address"=u16 4611, "values"=u16[] [1]) -> (w312:cluster{"starting address":u16, "values":u16[]})
        n227 = Enqueue Element(queue=w311, element=w312) -> ()  [unwired: 2 in, 3 out]
      }
      event "定时启动": Mouse Down {
        n228 = event-data() -> ()  [unwired: 1 in, 8 out]
        n229 = call "COD定时启动对话框.vi"() -> ("设置值"=→"设置值":dbl, "确定输出"=w315:bool)  [unwired: 10 in]
        n230 = local write "定时启动"(w315) -> ()
      }
      event "校准1", "校准2", "校准3", "校准4", "校准5", "校准6": Value Change {
        n231 = event-data() -> ()  [unwired: 1 in, 6 out]
        n232 = flat-sequence {
          tunnel: w319 -> [w322]
          tunnel: [w321] -> w318
          tunnel: [w320] -> w317
          tunnel: w318 -> [w359]
          tunnel: w317 -> [w358]
          frame #0 {
            n233 = Build Array("校准1", "校准2", "校准3", "校准4", "校准5", "校准6") -> (w323:bool[])
            n234 = for {
              tunnel: w323 -> [w340] mode=indexing
              tunnel: w322 -> [w336]
              tunnel: [w332] -> w321
              tunnel: [w331] -> w320
              i -> [w330]
              n235 = case shown="3" w330 {
                tunnel: ["浓度1" "浓度2" "浓度3" "浓度4" "浓度5" "浓度6"] -> w335
                frame 0, Default {
                }
                frame 1 {
                }
                frame 2 {
                }
                frame 3 {
                }
                frame 4 {
                }
                frame 5 {
                }
              }
              n236 = Multiply(x=w335, y=100.0) -> (x*y=w333:dbl)
              n237 = Insert Into Array(array=u16[] [] ("values"), index=0 ("索引"), new element=w333) -> (w337:u16[])
              n238 = case shown="真" w340 {
                tunnel: w337 -> [_ w353]
                tunnel: w336 -> [w347 w352]
                tunnel: [w347 w351] -> w332
                tunnel: [_ w350] -> w331
                tunnel: w330 -> [_ w349]
                frame False {
                }
                frame True {
                  n239 = Increment(x=w349) -> (x+1=→"当前选用的校准":i32)
                  n240 = Bundle By Name(cluster=cluster{"starting address":u16, "values":u16[]} {"starting address"=4272, "values"=[]}, "starting address"=u16 4274, "values"=w353) -> (w355:cluster{"starting address":u16, "values":u16[]})
                  n241 = Enqueue Element(queue=w352, element=w355) -> (queue out=w351:refnum<queue>, error out=w350:errorcluster)  [unwired: 2 in, 1 out]
                }
              }
            }
          }
          frame #1 {
            n242 = local read "当前选用的校准"() -> (w364:i32)
            n243 = case shown="4" w364 {
              tunnel: [w370 w371 w372 w373 w374 w375] -> w363
              frame 1, Default {
                n244 = local read "浓度1"() -> (w370:dbl)
              }
              frame 2 {
                n245 = local read "浓度2"() -> (w371:dbl)
              }
              frame 3 {
                n246 = local read "浓度3"() -> (w372:dbl)
              }
              frame 4 {
                n247 = local read "浓度4"() -> (w373:dbl)
              }
              frame 5 {
                n248 = local read "浓度5"() -> (w374:dbl)
              }
              frame 6 {
                n249 = local read "浓度6"() -> (w375:dbl)
              }
            }
            n250 = Not Equal To 0?(x=w363) -> (x != 0?=w362:bool)
            n251 = case shown="真" w362 {
              tunnel: [u16 8 ("address") u16 9 ("address")] -> w367
              tunnel: ["校零" ("测量模式") "校标" ("测量模式")] -> w357
              frame False {
              }
              frame True {
              }
            }
            n252 = global write "COD测量模式全局.vi" "测量模式"(w357) -> ()
            n253 = Insert Into Array(array=u16[] [] ("values"), index=0 ("索引"), new element=w367) -> (w361:u16[])
            n254 = Bundle By Name(cluster=cluster{"starting address":u16, "values":u16[]} {"starting address"=0, "values"=[]}, "starting address"=u16 4608 ("address"), "values"=w361) -> (w369:cluster{"starting address":u16, "values":u16[]})
            n255 = Enqueue Element(queue=w359, element=w369, error in (no error)=w358) -> ()  [unwired: 1 in, 3 out]
          }
          frame #2 {
            n256 = local write "枚举"(enum16{"读取数据", "写入数据", "读取写入DATABASE", "读取参数"}."写入数据" ("枚举")) -> ()
            n257 = call <vilib>:"Application Directory.vi"() -> ("Application Directory"=w387:path)
            n258 = Build Path(base path=w387, name or relative path="data\\Set.ini" ("名称或相对路径")) -> (appended path=w389:path)
            n259 = local read "当前选用的校准"() -> (w382:i32)
            n260 = call <vilib>:"Open Config Data.vi"("configuration file path"=w389) -> ("error out"=w385:errorcluster, "refnum"=w386:T10)  [unwired: 8 in, 1 out]
            n261 = call-poly <vilib>:"Write Key.vi"("section"="CODMn", "error in (no error)"=w385, "value"=w382, "key"="当前选用的校准" ("section"), "refnum"=w386) -> ("error out"=w380:errorcluster, "refnum out"=w381:T10)  [unwired: 4 in, 1 out]
            n262 = call <vilib>:"Close Config Data.vi"("error in (no error)"=w380, "refnum"=w381) -> ()  [unwired: 8 in, 2 out]
          }
        }
      }
      event "浓度1", "浓度2", "浓度3", "泵滴定数1", "泵滴定数2", "泵滴定数3", "浓度4", "浓度5", "浓度6", "泵滴定数4", "泵滴定数5", "泵滴定数6", "启用1", "启用2", "启用3", "启用4", "启用5", "启用6": Value Change {
        w392 = "CODMn" ("section")
        n263 = event-data() -> ()  [unwired: 1 in, 6 out]
        n264 = call <vilib>:"Application Directory.vi"() -> ("Application Directory"=w468:path)
        n265 = Build Path(base path=w468, name or relative path="data\\Set.ini" ("名称或相对路径")) -> (appended path=w466:path)
        n266 = call <vilib>:"Open Config Data.vi"("configuration file path"=w466) -> ("error out"=w464:errorcluster, "refnum"=w465:T10)  [unwired: 8 in, 1 out]
        n267 = local read "浓度1"() -> (w462:dbl)
        n268 = local read "浓度2"() -> (w446:dbl)
        n269 = call-poly <vilib>:"Write Key.vi"("section"=w392, "error in (no error)"=w464, "value"=w462, "key"="浓度1", "refnum"=w465) -> ("error out"=w461:errorcluster, "refnum out"=w460:T10)  [unwired: 4 in, 1 out]
        n270 = local read "浓度3"() -> (w436:dbl)
        n271 = call-poly <vilib>:"Write Key.vi"("section"=w392, "error in (no error)"=w461, "value"=w446, "key"="浓度2", "refnum"=w460) -> ("error out"=w459:errorcluster, "refnum out"=w458:T10)  [unwired: 4 in, 1 out]
        n272 = local read "泵滴定数1"() -> (w434:dbl)
        n273 = call-poly <vilib>:"Write Key.vi"("section"=w392, "error in (no error)"=w459, "value"=w436, "key"="浓度3", "refnum"=w458) -> ("error out"=w457:errorcluster, "refnum out"=w456:T10)  [unwired: 4 in, 1 out]
        n274 = call-poly <vilib>:"Write Key.vi"("section"=w392, "error in (no error)"=w457, "value"=w434, "key"="泵滴定数1", "refnum"=w456) -> ("error out"=w455:errorcluster, "refnum out"=w454:T10)  [unwired: 4 in, 1 out]
        n275 = local read "泵滴定数2"() -> (w432:dbl)
        n276 = call-poly <vilib>:"Write Key.vi"("section"=w392, "error in (no error)"=w455, "value"=w432, "key"="泵滴定数2", "refnum"=w454) -> ("error out"=w453:errorcluster, "refnum out"=w452:T10)  [unwired: 4 in, 1 out]
        n277 = local read "泵滴定数3"() -> (w430:dbl)
        n278 = local read "浓度4"() -> (w428:dbl)
        n279 = call-poly <vilib>:"Write Key.vi"("section"=w392, "error in (no error)"=w453, "value"=w430, "key"="泵滴定数3", "refnum"=w452) -> ("error out"=w451:errorcluster, "refnum out"=w450:T10)  [unwired: 4 in, 1 out]
        n280 = local read "浓度5"() -> (w425:dbl)
        n281 = call-poly <vilib>:"Write Key.vi"("section"=w392, "error in (no error)"=w451, "value"=w428, "key"="浓度4", "refnum"=w450) -> ("error out"=w444:errorcluster, "refnum out"=w445:T10)  [unwired: 4 in, 1 out]
        n282 = local read "浓度6"() -> (w424:dbl)
        n283 = call-poly <vilib>:"Write Key.vi"("section"=w392, "error in (no error)"=w444, "value"=w425, "key"="浓度5", "refnum"=w445) -> ("error out"=w443:errorcluster, "refnum out"=w442:T10)  [unwired: 4 in, 1 out]
        n284 = call-poly <vilib>:"Write Key.vi"("section"=w392, "error in (no error)"=w443, "value"=w424, "key"="浓度6", "refnum"=w442) -> ("error out"=w440:errorcluster, "refnum out"=w441:T10)  [unwired: 4 in, 1 out]
        n285 = local read "泵滴定数4"() -> (w422:dbl)
        n286 = call-poly <vilib>:"Write Key.vi"("section"=w392, "error in (no error)"=w440, "value"=w422, "key"="泵滴定数4", "refnum"=w441) -> ("error out"=w449:errorcluster, "refnum out"=w448:T10)  [unwired: 4 in, 1 out]
        n287 = local read "泵滴定数5"() -> (w420:dbl)
        n288 = call-poly <vilib>:"Write Key.vi"("section"=w392, "error in (no error)"=w449, "value"=w420, "key"="泵滴定数5", "refnum"=w448) -> ("error out"=w438:errorcluster, "refnum out"=w439:T10)  [unwired: 4 in, 1 out]
        n289 = local read "泵滴定数6"() -> (w418:dbl)
        n290 = local read "启用1"() -> (w408:bool)
        n291 = call-poly <vilib>:"Write Key.vi"("section"=w392, "error in (no error)"=w438, "value"=w418, "key"="泵滴定数6", "refnum"=w439) -> ("error out"=w417:errorcluster, "refnum out"=w416:T10)  [unwired: 4 in, 1 out]
        n292 = local read "启用2"() -> (w405:bool)
        n293 = call-poly <vilib>:"Write Key.vi"("section"=w392, "error in (no error)"=w417, "value"=w408, "key"="启用1", "refnum"=w416) -> ("error out"=w404:errorcluster, "refnum out"=w407:T10)  [unwired: 4 in, 1 out]
        n294 = call-poly <vilib>:"Write Key.vi"("section"=w392, "error in (no error)"=w404, "value"=w405, "key"="启用2", "refnum"=w407) -> ("error out"=w415:errorcluster, "refnum out"=w414:T10)  [unwired: 4 in, 1 out]
        n295 = local read "启用3"() -> (w403:bool)
        n296 = local read "启用4"() -> (w401:bool)
        n297 = call-poly <vilib>:"Write Key.vi"("section"=w392, "error in (no error)"=w415, "value"=w403, "key"="启用3", "refnum"=w414) -> ("error out"=w413:errorcluster, "refnum out"=w412:T10)  [unwired: 4 in, 1 out]
        n298 = local read "启用5"() -> (w398:bool)
        n299 = call-poly <vilib>:"Write Key.vi"("section"=w392, "error in (no error)"=w413, "value"=w401, "key"="启用4", "refnum"=w412) -> ("error out"=w411:errorcluster, "refnum out"=w410:T10)  [unwired: 4 in, 1 out]
        n300 = call-poly <vilib>:"Write Key.vi"("section"=w392, "error in (no error)"=w411, "value"=w398, "key"="启用5", "refnum"=w410) -> ("error out"=w396:errorcluster, "refnum out"=w395:T10)  [unwired: 4 in, 1 out]
        n301 = local read "启用6"() -> (w397:bool)
        n302 = call-poly <vilib>:"Write Key.vi"("section"=w392, "error in (no error)"=w396, "value"=w397, "key"="启用6", "refnum"=w395) -> ("error out"=w393:errorcluster, "refnum out"=w394:T10)  [unwired: 4 in, 1 out]
        n303 = call <vilib>:"Close Config Data.vi"("error in (no error)"=w393, "refnum"=w394) -> ()  [unwired: 8 in, 2 out]
      }
      event "读取": Value Change {
        n304 = event-data() -> ()  [unwired: 1 in, 6 out]
        n305 = local write "枚举"(enum16{"读取数据", "写入数据", "读取写入DATABASE", "读取参数"}."读取参数" ("枚举")) -> ()
        n306 = Bundle By Name(cluster=T7 {"starting address"=0, "number of holding registers"=0}, "starting address"=u16 4616, "number of holding registers"=u16 8) -> (w478:T7)
        n307 = Flush Queue(queue=w471, error in (no error)=w470) -> (queue out=w474:refnum<queue>, error out=w473:errorcluster)  [unwired: 1 out]
        n308 = Enqueue Element(queue=w474, element=w478, error in (no error)=w473) -> ()  [unwired: 1 in, 3 out]
        "读取KB值" <- TRUE
      }
      event "方程参数写入": Value Change {
        n309 = event-data() -> ()  [unwired: 1 in, 6 out]
        n310 = flat-sequence {
          tunnel: w479 -> [w489]
          frame #0 {
            n311 = local read "b 2"() -> (w482:dbl)
            n312 = local read "K 2"() -> (w483:dbl)
            n313 = local read "b"() -> (w484:dbl)
            n314 = local read "K"() -> (w485:dbl)
            n315 = Build Array(w485, w484, w483, w482) -> (w481:dbl[])
            n316 = call "浮点转CDAB整形cod.vi"("浮点数"=w481) -> ("CDAB整形输出"=w480:u16[])  [unwired: 10 in]
            n317 = Bundle By Name(cluster=cluster{"starting address":u16, "values":u16[]} {"starting address"=4272, "values"=[]}, "starting address"=u16 4616 ("address"), "values"=w480) -> (w491:cluster{"starting address":u16, "values":u16[]})
            n318 = Enqueue Element(queue=w489, element=w491, timeout in ms (-1)=1000 ("超时毫秒(-1)")) -> (error out=w486:errorcluster)  [unwired: 1 in, 2 out]
            n319 = case shown="错误" w486 {
              tunnel: ["写入成功" ("消息") "写入失败" ("消息")] -> w487
              frame No Error {
              }
              frame Error {
              }
            }
            n320 = One Button Dialog(message=w487) -> ()  [unwired: 1 in, 1 out]
          }
          frame #1 {
            n321 = local write "枚举"(enum16{"读取数据", "写入数据", "读取写入DATABASE", "读取参数"}."写入数据" ("枚举")) -> ()
          }
        }
      }
      event "读取方程系数.写入": Value Change {
        n322 = event-data() -> ()  [unwired: 1 in, 6 out]
        n323 = flat-sequence {
          tunnel: w496 -> [w509]
          frame #0 {
            n324 = Unbundle By Name("读取方程系数") -> ("k"=w503:dbl, "b"=w502:dbl, "k 2"=w498:dbl, "b 2"=w497:dbl)
            n325 = Bundle By Name(cluster=cluster{"k":dbl, "b":dbl, "k 2":dbl, "b 2":dbl} {"k"=0.0, "b"=0.0, "k 2"=0.0, "b 2"=0.0} ("读取方程系数 2"), "k"=w503, "b"=w502, "k 2"=w498, "b 2"=w497) -> (w501:cluster{"k":dbl, "b":dbl, "k 2":dbl, "b 2":dbl})
            n326 = Cluster To Array(cluster=w501) -> (array=w505:dbl[])
            n327 = call "浮点转CDAB整形cod.vi"("浮点数"=w505) -> ("CDAB整形输出"=w500:u16[])  [unwired: 10 in]
            n328 = Bundle By Name(cluster=cluster{"starting address":u16, "values":u16[]} {"starting address"=4272, "values"=[]}, "starting address"=u16 4616 ("address"), "values"=w500) -> (w511:cluster{"starting address":u16, "values":u16[]})
            n329 = Enqueue Element(queue=w509, element=w511, timeout in ms (-1)=1000 ("超时毫秒(-1)")) -> (error out=w506:errorcluster)  [unwired: 1 in, 2 out]
            n330 = case shown="错误" w506 {
              tunnel: ["写入成功" ("消息") "写入失败" ("消息")] -> w507
              frame No Error {
              }
              frame Error {
              }
            }
            n331 = One Button Dialog(message=w507) -> ()  [unwired: 1 in, 1 out]
          }
          frame #1 {
            n332 = local write "枚举"(enum16{"读取数据", "写入数据", "读取写入DATABASE", "读取参数"}."写入数据" ("枚举")) -> ()
          }
        }
      }
    }
  }
  n333 = while {
    tunnel: w20 -> [w647]
    tunnel: w19 -> [w646]
    tunnel: w8 -> [w641]
    tunnel: w7 -> [w640]
    i -> [w642]
    stop <- FALSE stop-if-true
    w533 = T12 0 items=["最小二乘", "最小绝对残差", "Bisquare"] ("method")
    w529 = T12 0 items=["最小二乘", "最小绝对残差", "Bisquare"] ("method")
    # "自动校时"
    n334 = Multiply(x="浓度 2", y=100.0) -> (x*y=w611:dbl)
    n335 = Build Array("启用1", "启用2", "启用3") -> (w573:bool[])
    n336 = local read "启用3"() -> (w527:bool)
    n337 = Multiply(x="温度", y=10.0) -> (x*y=w614:dbl)
    n338 = local read "泵滴定数3"() -> (w523:dbl)
    n339 = local read "泵滴定数1"() -> (w521:dbl)
    n340 = local read "泵滴定数2"() -> (w522:dbl)
    n341 = local read "启用2"() -> (w526:bool)
    n342 = local read "启用1"() -> (w525:bool)
    n343 = local read "启用6"() -> (w535:bool)
    n344 = Wait (ms)(milliseconds to wait=u32 1000 ("等待时间（毫秒）")) -> ()  [unwired: 1 out]
    n345 = local read "泵滴定数6"() -> (w539:dbl)
    n346 = local read "泵滴定数4"() -> (w541:dbl)
    n347 = local read "泵滴定数5"() -> (w540:dbl)
    n348 = local read "启用5"() -> (w536:bool)
    n349 = local read "启用4"() -> (w537:bool)
    n350 = Index Array(array=w573) -> (element #1=w572:bool, element #2=w569:bool, element #3=w566:bool)  [unwired: 3 in]
    n351 = local read "浓度2"() -> (w518:dbl)
    n352 = local read "浓度3"() -> (w519:dbl)
    n353 = local read "浓度1"() -> (w517:dbl)
    n354 = local write "浓度"(w611) -> ()
    n355 = local read "浓度5"() -> (w544:dbl)
    n356 = local read "浓度6"() -> (w543:dbl)
    n357 = local read "浓度4"() -> (w545:dbl)
    n358 = Bundle By Name(cluster=T7 {"starting address"=4224, "number of holding registers"=16}, "starting address"=u16 4224, "number of holding registers"=u16 50) -> (w704:T7)
    n359 = local write "温度 2"(w614) -> ()
    n360 = case shown="真" "启用6" {
      tunnel: [w726 w728] -> w556
      tunnel: [w725 w727] -> w555
      frame False {
        n361 = local read "泵滴定数4"() -> (w726:dbl)
        n362 = local read "浓度4"() -> (w725:dbl)
      }
      frame True {
        n363 = local read "泵滴定数6"() -> (w728:dbl)
        n364 = local read "浓度6"() -> (w727:dbl)
      }
    }
    n365 = Multiply(x="修正系数 2", y=100.0) -> (x*y=w608:dbl)
    n366 = case shown="假" "启用5" {
      tunnel: [w730 w732] -> w560
      tunnel: [w729 w731] -> w559
      frame False {
        n367 = local read "泵滴定数6"() -> (w730:dbl)
        n368 = local read "浓度6"() -> (w729:dbl)
      }
      frame True {
        n369 = local read "泵滴定数5"() -> (w732:dbl)
        n370 = local read "浓度5"() -> (w731:dbl)
      }
    }
    n371 = case shown="假" "启用4" {
      tunnel: [w734 w736] -> w563
      tunnel: [w733 w735] -> w562
      frame False {
        n372 = local read "泵滴定数5"() -> (w734:dbl)
        n373 = local read "浓度5"() -> (w733:dbl)
      }
      frame True {
        n374 = local read "泵滴定数4"() -> (w736:dbl)
        n375 = local read "浓度4"() -> (w735:dbl)
      }
    }
    n376 = case shown="假" w566 {
      tunnel: [w737 w740] -> w565
      tunnel: [w738 w739] -> w564
      frame False {
        n377 = local read "泵滴定数1"() -> (w737:dbl)
        n378 = local read "浓度1"() -> (w738:dbl)
      }
      frame True {
        n379 = local read "泵滴定数3"() -> (w740:dbl)
        n380 = local read "浓度3"() -> (w739:dbl)
      }
    }
    n381 = case shown="真" w572 {
      tunnel: [w746 w748] -> w571
      tunnel: [w745 w747] -> w570
      frame False {
        n382 = local read "泵滴定数2"() -> (w746:dbl)
        n383 = local read "浓度2"() -> (w745:dbl)
      }
      frame True {
        n384 = local read "泵滴定数1"() -> (w748:dbl)
        n385 = local read "浓度1"() -> (w747:dbl)
      }
    }
    n386 = case shown="假" w569 {
      tunnel: [w742 w744] -> w568
      tunnel: [w741 w743] -> w567
      frame False {
        n387 = local read "泵滴定数3"() -> (w742:dbl)
        n388 = local read "浓度3"() -> (w741:dbl)
      }
      frame True {
        n389 = local read "泵滴定数2"() -> (w744:dbl)
        n390 = local read "浓度2"() -> (w743:dbl)
      }
    }
    n391 = Build Array(w525, w526, w527) -> (w528:bool[])
    n392 = Build Array(w537, w536, w535) -> (w534:bool[])
    n393 = local write "修正系数"(w608) -> ()
    n394 = Build Array(w517, w518, w519) -> (w520:dbl[])
    n395 = Build Array(w521, w522, w523) -> (w524:dbl[])
    n396 = Build Array(w545, w544, w543) -> (w542:dbl[])
    n397 = Build Array(w541, w540, w539) -> (w538:dbl[])
    n398 = call "线性公式CODMn用.vi"("精度"=4, "模型"=enum32{"线性", "多项式"}."线性", "method"=w529, "启用"=w528, "监测浓度"=w524, "标液浓度"=w520) -> ("拟合方程"=→"低量程拟合方程":string)  [unwired: 3 in, 2 out]
    n399 = call "线性公式CODMn用.vi"("精度"=4, "模型"=enum32{"线性", "多项式"}."线性", "method"=w533, "启用"=w534, "监测浓度"=w538, "标液浓度"=w542) -> ("拟合方程"=→"高量程拟合方程":string)  [unwired: 3 in, 2 out]
    n400 = formula code="float x,y,g,h,k,b;\nx=(x1+x2+x3)/3;\ny=(y1+y2+y3)/3;\ng=(x1-x)*(y1-y)+(x2-x)*(y2-y)+(x3-x)*(y3-y);\nh=pow((x1-x),2)+pow((x2-x),2)+pow((x3-x),2);\nk=g/h;\nb=y-k*x;"("x1"=w563, "x2"=w560, "x3"=w556, "y1"=w562, "y2"=w559, "y3"=w555) -> ("k"=→"K 2":dbl, "b"=→"b 2":dbl)
    n401 = formula code="float x,y,g,h,k,b;\nx=(x1+x2+x3)/3;\ny=(y1+y2+y3)/3;\ng=(x1-x)*(y1-y)+(x2-x)*(y2-y)+(x3-x)*(y3-y);\nh=pow((x1-x),2)+pow((x2-x),2)+pow((x3-x),2);\nk=g/h;\nb=y-k*x;"("x1"=w571, "x2"=w568, "x3"=w565, "y1"=w570, "y2"=w567, "y3"=w564) -> ("k"=→"K":dbl, "b"=→"b":dbl)
    n402 = Enqueue Element(queue=w647, element=w704, error in (no error)=w646) -> ()  [unwired: 1 in, 3 out]
    n403 = local read "Registers"() -> (w698:u16[])
    n404 = Index Array(array=w698, index #1=0 ("索引"), index #4=3 ("索引"), index #14=13 ("索引"), index #15=14 ("索引"), index #32=31 ("索引")) -> (element #1=w605:u16, element #2=w604:u16, element #3=w603:u16, element #4=w549:u16, element #5=→"模式（受控）":u16, element #6=→"进样管":u16, element #7=→"高锰酸钾":u16, element #8=→"草酸钠":u16, element #9=→"硫酸":u16, element #10=→"ORP显示":u16, element #11=w675:u16, element #12=w677:u16, element #13=w690:u16, element #14=w694:u16, element #15=w649:u16, element #16=w602:u16, element #33=→"分":u16, element #34=→"秒":u16)  [unwired: 29 in, 16 out]
    "多列列表框" <- w602
    n405 = global write "运行时序全局变量.vi" "多列列表框"(w602) -> ()
    n406 = Divide(x=w694, y=u16 1000) -> (x/y=→"零点滴定值":dbl)
    n407 = Divide(x=w649, y=u16 1000) -> (x/y=→"标度滴定值":dbl)
    n408 = feedback #1(w602) -> (w621:u16)
    n409 = feedback-in #1(w602) -> ()
    n410 = Build Array(w605, w604, w603) -> (w606:u16[])
    n411 = Equal?(x=w677, y=u16 1) -> (x = y?=→"排液标记":bool)
    n412 = Equal?(x=w549, y=u16 0) -> (x = y?=→"待机":bool)
    n413 = Equal?(x=w549, y=u16 7) -> (x = y?=→"质控样测量":bool)
    n414 = Equal?(x=w549, y=u16 1) -> (x = y?=→"水样测量":bool)
    n415 = Equal?(x=w602, y=u16 5) -> (x = y?=w645:bool)
    n416 = Equal?(x=w549, y=u16 9) -> (x = y?=→"校标标记":bool)
    n417 = Equal?(x=w549, y=u16 6) -> (x = y?=→"平行样测量":bool)
    n418 = Equal?(x=w549, y=u16 2) -> (x = y?=→"标样核查标记":bool)
    n419 = Equal?(x=w549, y=u16 8) -> (x = y?=→"校零标记":bool)
    n420 = Equal?(x=w690, y=u16 1) -> (x = y?=w638:bool)
    "ORP故障" <- w638
    n421 = Equal?(x=w690, y=u16 2) -> (x = y?=w637:bool)
    "温控器故障" <- w637
    n422 = Equal?(x=w690, y=u16 3) -> (x = y?=w636:bool)
    "加热故障" <- w636
    n423 = Equal?(x=w690, y=u16 4) -> (x = y?=w635:bool)
    "高锰酸钾报警" <- w635
    n424 = Equal?(x=w690, y=u16 5) -> (x = y?=w634:bool)
    "草酸钠报警" <- w634
    n425 = Equal?(x=w690, y=u16 6) -> (x = y?=w633:bool)
    "测量错误" <- w633
    n426 = Equal?(x=w690, y=u16 8) -> (x = y?=w632:bool)
    "校零错误" <- w632
    n427 = Equal?(x=w690, y=u16 7) -> (x = y?=w631:bool)
    "校标错误" <- w631
    n428 = Equal?(x=w690, y=u16 9) -> (x = y?=w630:bool)
    "进水样超量程" <- w630
    n429 = Divide(x=w675, y=u16 10) -> (x/y=→"温度":dbl)
    n430 = Equal?(x=w549, y=u16 10) -> (x = y?=→"加标回收测量":bool)
    n431 = Equal?(x=w690, y=u16 10) -> (x = y?=w629:bool)
    "排液故障" <- w629
    n432 = Equal?(x=w549, y=u16 3) -> (x = y?=→"零点核查标记":bool)
    n433 = Compound Arithmetic op=OR ("复合运算")(w638, w637, w636, w635, w634, w633, w631, w632, w630, w629) -> (→"故障标记":bool)
    n434 = Not Equal?(x=w602, y=w621) -> (x != y?=w620:bool)
    n435 = call <vilib>:"Boolean Crossing PtByPt.vi"("direction"=enum16{"either", "false-true", "true-false"}."false-true", "input"=w645) -> ("crossing"=w643:bool)  [unwired: 1 in]
    n436 = Bundle By Name(cluster=T4 {"ORP故障"=FALSE, "温控器故障"=FALSE, "加热故障"=FALSE, "高锰酸钾报警"=FALSE, "草酸钠报警"=FALSE, "测量错误"=FALSE, "校零错误"=FALSE, "校标错误"=FALSE, " 进水样超量程"=FALSE, "排液阀故障"=FALSE} ("报警簇"), "ORP故障"=w638, "温控器故障"=w637, "加热故障"=w636, "高锰酸钾报警"=w635, "草酸钠报警"=w634, "测量错误"=w633, "校零错误"=w632, "校标错误"=w631, "进水样超量程"=w630, "排液阀故障"=w629) -> (w622:T4)
    "报警簇" <- w622
    n437 = call "HexToDate.vi"("数组"=w606) -> ("DATE"=w600:timestamp[])  [unwired: 10 in]
    n438 = case shown="真" w643 {
      tunnel: w641 -> [_ w822]
      tunnel: w640 -> [_ w817]
      frame False {
      }
      frame True {
        n439 = Bundle By Name(cluster=T7 {"starting address"=0, "number of holding registers"=0}, "starting address"=u16 4101, "number of holding registers"=u16 10) -> (w821:T7)
        n440 = Enqueue Element(queue=w822, element=w821, error in (no error)=w817) -> ()  [unwired: 1 in, 3 out]
        n441 = local write "枚举"(enum16{"读取数据", "写入数据", "读取写入DATABASE", "读取参数"}."读取写入DATABASE" ("枚举")) -> ()
      }
    }
    n442 = case shown="真" w620 {
      tunnel: w602 -> [_ w800]
      frame False {
      }
      frame True {
        n443 = property on="多列列表框" class="MCListbox (严格)"() -> ("ItemNames"=w794:string[][])  [unwired: 2 in, 2 out]
        n444 = Index Array(array=w794, index (row)=w800) -> (element=w791:string[])  [unwired: 1 in]
        n445 = Index Array(array=w791, index=0 ("索引")) -> (element=w789:string)
        n446 = Array To Spreadsheet String(delimiter (Tab)="-" ("分隔符(Tab)"), array=w791, 3:"" ("格式字符串")) -> ()  [unwired: 1 out]
        n447 = Get Date/Time In Seconds() -> (seconds since 1Jan1904=w798:timestamp)
        n448 = Bundle(cluster="data in", "时间标识"=w798, "参数"="CODMn" ("table输入"), "日志信息"=w789, "流程参数"="" ("table输入")) -> (w795:T3)
        n449 = call "流程日志字段定义.vi"("table输入"="操作日志", "data in"=w795) -> ("table输出"=w803:string, "columns"=w804:string[], "data out"=w805:T13)  [unwired: 7 in]
        n450 = call "插入数据.vi"("data"=w805, "columns"=w804, "database"="database3.mdb", "table"=w803) -> ()  [unwired: 7 in, 1 out]
      }
    }
    n451 = Index Array(array=w600) -> (element=→"仪器时间":timestamp)  [unwired: 1 in]
    n452 = Get Date/Time In Seconds() -> (seconds since 1Jan1904=w599:timestamp)
    "系统时间" <- w599
    n453 = disable-structure shown="禁用" {
      frame Disabled {
        n454 = local read "标样核查标记"() -> (w713:bool)
        n455 = local read "零点核查标记"() -> (w712:bool)
        n456 = local read "加标回收测量"() -> (w711:bool)
        n457 = local read "平行样测量"() -> (w710:bool)
        n458 = local read "水样测量"() -> (w714:bool)
        n459 = local read "校零标记"() -> (w709:bool)
        n460 = local read "校标标记"() -> (w708:bool)
        n461 = Build Array(w714, w713, w712, w711, w710, w709, w708) -> (w707:bool[])
        n462 = for {
          tunnel: w707 -> [w723] mode=indexing
          i -> [w722]
          n463 = case shown="真" w723 {
            tunnel: w722 -> [_ w724]
            frame False {
            }
            frame True {
              "测量模式数字" <- w724
            }
          }
        }
        n464 = local read "测量模式数字"() -> (w706:i32)
        n465 = case shown="0, 默认" w706 {
          tunnel: ["水样测试" ("测量模式") "标样核查" ("测量模式") "零点核查" ("测量模式") "加标回收" ("测量模式") "平行样" ("测量模式") "校零" ("测量模式") "校标" ("测量模式")] -> w705
          frame 0, Default {
          }
          frame 1 {
          }
          frame 2 {
          }
          frame 3 {
          }
          frame 4 {
          }
          frame 5 {
          }
          frame 6 {
          }
        }
        n466 = global write "COD测量模式全局.vi" "测量模式"(w705) -> ()
      }
      frame Enabled {
      }
    }
    n467 = global read "COD读取DATA全局.vi" "data"() -> (w582:T6)
    n468 = global read "COD测量模式全局.vi" "测量模式"() -> (w581:string)
    n469 = Build Array(w599) -> (w598:timestamp[])
    n470 = Unbundle By Name(w582) -> ("时间"=w579:timestamp, "检测值"=w578:sgl, "数据标识"=w577:string)
    n471 = call "DateToHex.vi"("DATE"=w598) -> ("数组"=w597:u16[])  [unwired: 10 in]
    n472 = call "DateToHex.vi"("DATE"=w600) -> ("数组"=w592:u16[])  [unwired: 10 in]
    n473 = local read "测量数据区"() -> (w583:T2)
    n474 = case shown="\"水样测试\"" w581 {
      tunnel: w583 -> [w749 w754 w759 w764 w769 w774 w779 w784]
      tunnel: [w749 w753 w755 w763 w768 w773 w775 w783] -> w580
      tunnel: w579 -> [_ w752 w758 w762 w767 w772 w778 w782]
      tunnel: w578 -> [_ w751 w757 w761 w766 w771 w777 w781]
      tunnel: w577 -> [_ w750 w756 w760 w765 w770 w776 w780]
      frame "", Default {
      }
      frame "水样测试" {
        n475 = Bundle By Name(cluster=w754, "水样数据时间"=w752, "水样实测值"=w751, "水样数据标识"=w750) -> (w753:T2)
      }
      frame "标样核查" {
        n476 = Bundle By Name(cluster=w759, "跨度核查数据时间"=w758, "跨度核查实测值"=w757, "跨度核查数据标识"=w756) -> (w755:T2)
      }
      frame "零点核查" {
        n477 = Bundle By Name(cluster=w764, "零点核查数据时间"=w762, "零点核查实测值"=w761, "零点核查数据标识"=w760) -> (w763:T2)
      }
      frame "加标回收" {
        n478 = Bundle By Name(cluster=w769, "加标回收数据时间"=w767, "加标回收实测值"=w766, "加标回收数据标识"=w765) -> (w768:T2)
      }
      frame "平行样" {
        n479 = Bundle By Name(cluster=w774, "平行样数据时间"=w772, "平行样实测值"=w771, "平行样数据标识"=w770) -> (w773:T2)
      }
      frame "校零" {
        n480 = Bundle By Name(cluster=w779, "空白数据时间"=w778, "空白实测值"=w777, "空白数据标识"=w776) -> (w775:T2)
      }
      frame "校标" {
        n481 = Bundle By Name(cluster=w784, "标样数据时间"=w782, "标样实测值"=w781, "标样数据标识"=w780) -> (w783:T2)
      }
    }
    "测量数据区" <- w580
    n482 = Index Array(array=w592, index=2 ("索引")) -> (element=w594:u16)
    n483 = Index Array(array=w597, index=2 ("索引")) -> (element=w595:u16)
    n484 = Split Number(x=w594) -> (hi(x)=w588:u8)  [unwired: 1 out]
    n485 = call "CODMn报警信息.vi"("报警簇"=w622) -> ("CODMN报警信息"=w623:string)  [unwired: 10 in]
    n486 = Split Number(x=w595) -> (hi(x)=w591:u8)  [unwired: 1 out]
    n487 = To Byte Integer(number=w588) -> (8bit integer=w587:i8)
    n488 = To Byte Integer(number=w591) -> (8bit integer=w590:i8)
    n489 = Subtract(x=w587, y=w590) -> (x-y=w589:i8)
    n490 = feedback #2(w623) -> (w624:string)
    n491 = feedback-in #2(w623) -> ()
    n492 = Not Equal?(x=w623, y="") -> (x != y?=w628:bool)
    n493 = Absolute Value(x=w589) -> (abs(x)=w586:i8)
    n494 = Greater Or Equal?(x=w586, y=i8 5) -> (x >= y?=w584:bool)
    n495 = Not Equal?(x=w623, y=w624) -> (x != y?=w625:bool)
    n496 = case shown="真" w584 {
      tunnel: w584 -> [_ w785]
      frame False {
      }
      frame True {
        n497 = flat-sequence {
          tunnel: w785 -> [_]
          frame #0 {
            n498 = property on="时间校准" class="Bool (严格)"("Val(Sgnl)"=TRUE ("时间校准")) -> ()  [unwired: 2 in, 2 out]
          }
          frame #1 {
            n499 = Wait (ms)(milliseconds to wait=u32 300 ("等待时间（毫秒）")) -> ()  [unwired: 1 out]
          }
          frame #2 {
            n500 = property on="时间校准" class="Bool (严格)"("Val(Sgnl)"=FALSE ("时间校准")) -> ()  [unwired: 2 in, 2 out]
          }
        }
      }
    }
    n501 = And(x=w625, y=w628) -> (x .and. y?=w626:bool)
    n502 = case shown="真" w626 {
      tunnel: w623 -> [_ w806]
      frame False {
      }
      frame True {
        n503 = Get Date/Time In Seconds() -> (seconds since 1Jan1904=w808:timestamp)
        n504 = Bundle By Name(cluster=T11 {"时间标识"=timestamp(0 s since 1904-01-01), "设备"="", "日志信息"=""} ("data in"), "时间标识"=w808, "设备"="CODMn", "日志信息"=w806) -> (w809:T11)
        n505 = call "报警信息字段定义.vi"("table输入"="报警信息", "data in"=w809) -> ("table输出"=w813:string, "columns"=w814:string[], "data out"=w815:T11)  [unwired: 7 in]
        n506 = call "插入数据.vi"("data"=w815, "columns"=w814, "database"="database3.mdb", "table"=w813) -> ()  [unwired: 7 in, 1 out]
      }
    }
    "循环次数" <- w642
  }
  n507 = while {
    tunnel: w1 -> [w824]
    stop <- FALSE stop-if-true
    n508 = event shown="[0] \"保存\": 鼠标按下" {
      selector: _ -> [_]
      dyn-events: _ -> [_]
      timeout: _ -> [_]
      tunnel: w824 -> [w834]
      event "保存": Mouse Down {
        n509 = event-data() -> ()  [unwired: 1 in, 8 out]
        n510 = local write "枚举"(enum16{"读取数据", "写入数据", "读取写入DATABASE", "读取参数"}."写入数据" ("枚举")) -> ()
        n511 = local write "恒温时间"("恒温时间") -> ()
        n512 = local write "标样浓度 2"("标样浓度 2") -> ()
        n513 = local write "修正系数"("修正系数") -> ()
        n514 = local write "加标回收"("加标回收") -> ()
        n515 = local write "水样"("水样") -> ()
        n516 = local write "标液"("标液") -> ()
        n517 = local write "硫酸"("硫酸") -> ()
        n518 = local write "高锰酸钾"("高锰酸钾") -> ()
        n519 = local write "零点泵计量数 2"("零点泵计量数 2") -> ()
        n520 = local write "标度泵计量数 2"("标度泵计量数 2") -> ()
        n521 = local write "基本量程"("基本量程") -> ()
        n522 = local write "蒸馏水"("蒸馏水") -> ()
        n523 = local write "温度 2"("温度 2") -> ()
        n524 = local write "草酸钠"("草酸钠") -> ()
        n525 = local write "质控样"("质控样") -> ()
        n526 = Build Array("温度 2", "恒温时间", "浓度", "修正系数", "基本量程", "水样", "蒸馏水", "标液", "质控样", "加标回收", "高锰酸钾", "草酸钠", "硫酸", "零点泵计量数 2", "标度泵计量数 2", "标样浓度 2") -> (w832:dbl[])
        n527 = Bundle By Name(cluster=cluster{"starting address":u16, "values":u16[]} {"starting address"=4272, "values"=[]}, "starting address"=u16 4272, "values"=w832) -> (w830:cluster{"starting address":u16, "values":u16[]})
        n528 = Enqueue Element(queue=w834, element=w830, timeout in ms (-1)=1000 ("超时毫秒(-1)")) -> ()  [unwired: 1 in, 3 out]
      }
    }
  }
  n529 = while {
    tunnel: w5 -> [w865]
    tunnel: w4 -> [w864]
    tunnel: w1 -> [w863]
    tunnel: w20 -> [w862]
    tunnel: w19 -> [w861]
    tunnel: [w851] -> w18
    tunnel: [w860] -> w17
    tunnel: w13 -> [w858]
    tunnel: w12 -> [w857]
    tunnel: w8 -> [w856]
    tunnel: w7 -> [w855]
    tunnel: w6 -> [w854]
    tunnel: w1 -> [w848]
    i -> [w850]
    stop <- FALSE stop-if-true
    n530 = case shown="\"读取参数\"" "枚举" {
      tunnel: w865 -> [w915 w952 w1041 w1108]
      tunnel: w864 -> [w914 w948 w1040 w1107]
      tunnel: w863 -> [_ w951 _ _]
      tunnel: [w869 w950 w1043 w1102] -> w860
      tunnel: [w870 w949 w1042 w1100] -> w851
      tunnel: w862 -> [w912 _ _ _]
      tunnel: w861 -> [w908 _ _ _]
      tunnel: w858 -> [_ _ _ w1106]
      tunnel: w857 -> [_ _ _ w1105]
      tunnel: w856 -> [_ _ w1039 _]
      tunnel: w855 -> [_ _ w1038 _]
      tunnel: w854 -> [_ w947 _ _]
      tunnel: w848 -> [_ _ w985 _]
      frame "读取数据", Default {
        n531 = Dequeue Element(queue=w912, timeout in ms (-1)=1000 ("超时毫秒(-1)"), error in (no error)=w908) -> (element=w911:T7)  [unwired: 3 out]
        n532 = Unbundle By Name(w911) -> ("starting address"=w910:u16, "number of holding registers"=w909:u16)
        n533 = call <vilib>:"Read Holding Registers.vi"("error in (no error)"=w914, "quantity"=w909, "starting address"=w910, "MB session in"=w915) -> ("error out"=w903:errorcluster, "Registers"=→"Registers":u16[], "MB session out"=w906:refnum<class "MB_Master_Serial.lvclass">)  [unwired: 5 in]
        n534 = call <vilib>:"Read Coils.vi"("error in (no error)"=w903, "quantity"=u16 8, "starting address"=u16 140, "MB session in"=w906) -> ("error out"=w893:errorcluster, "Coils"=w902:bool[], "MB session out"=w894:refnum<class "MB_Master_Serial.lvclass">)  [unwired: 5 in]
        n535 = Index Array(array=w902) -> (element #1=→"进水样":bool, element #2=→"进蒸馏水":bool, element #3=→"进标液":bool, element #4=→"进质控样":bool, element #5=→"进加标回收样":bool, element #6=→"进高锰酸钾":bool, element #7=→"进草酸钠":bool, element #8=→"进硫酸":bool)  [unwired: 9 in, 1 out]
        n536 = call <vilib>:"Read Coils.vi"("error in (no error)"=w893, "quantity"=u16 1, "starting address"=u16 137, "MB session in"=w894) -> ("error out"=w889:errorcluster, "Coils"=w883:bool[], "MB session out"=w890:refnum<class "MB_Master_Serial.lvclass">)  [unwired: 5 in]
        n537 = Index Array(array=w883) -> (element=→"搅拌":bool)  [unwired: 1 in]
        n538 = call <vilib>:"Read Coils.vi"("error in (no error)"=w889, "quantity"=u16 1, "starting address"=u16 400, "MB session in"=w890) -> ("error out"=w871:errorcluster, "Coils"=w886:bool[], "MB session out"=w874:refnum<class "MB_Master_Serial.lvclass">)  [unwired: 5 in]
        n539 = Index Array(array=w886) -> (element=→"加热":bool)  [unwired: 1 in]
        n540 = call <vilib>:"Read Holding Registers.vi"("error in (no error)"=w871, "quantity"=u16 1 ("number of holding registers"), "starting address"=u16 4104, "MB session in"=w874) -> ("error out"=w870:errorcluster, "Registers"=w868:u16[], "MB session out"=w869:refnum<class "MB_Master_Serial.lvclass">)  [unwired: 5 in]
        n541 = property on="基本量程" class="Enum (严格)"() -> ("Value"=w878:enum16{"10mL", "20mL"})  [unwired: 2 in, 2 out]
        n542 = Index Array(array=w868) -> (element=w867:u16)  [unwired: 1 in]
        n543 = To Single Precision Float(number=w867) -> (single precision float=w880:sgl)
        n544 = Divide(x=w880, y=sgl 100.0) -> (x/y=w881:sgl)
        n545 = Less Or Equal?(x=w881, y=sgl 0.01) -> (x <= y?=w877:bool)
        n546 = case shown="真" w877 {
          tunnel: [w938 w940] -> w879
          tunnel: w881 -> [w938 _]
          frame False {
          }
          frame True {
            n547 = Increment(x=0.0) -> (x+1=w941:dbl)
            n548 = Divide(x=w941, y=sgl 100.0) -> (x/y=w940:dbl)
          }
        }
        n549 = case shown="\"20mL\"" w878 {
          tunnel: w879 -> [w918 w928]
          tunnel: [w916 w927] -> w866
          frame "10mL", Default {
            n550 = Less Or Equal?(x=w918, y=2.0) -> (x <= y?=w921:bool)
            n551 = Greater?(x=w918, y=0.0) -> (0:w920:bool)
            n552 = And(x=w921, y=w920) -> (x .and. y?=w917:bool)
            n553 = case shown="真" w917 {
              tunnel: w918 -> [w923 w926]
              tunnel: [w923 w924] -> w916
              frame False {
              }
              frame True {
                n554 = Multiply(x=w926, y=1.1) -> (x*y=w924:dbl)
              }
            }
          }
          frame "20mL" {
            n555 = Less Or Equal?(x=w928, y=4.0) -> (x <= y?=w932:bool)
            n556 = Greater?(x=w928, y=0.0) -> (0:w931:bool)
            n557 = And(x=w932, y=w931) -> (x .and. y?=w929:bool)
            n558 = case shown="真" w929 {
              tunnel: w928 -> [w934 w937]
              tunnel: [w934 w935] -> w927
              frame False {
              }
              frame True {
                n559 = Multiply(x=w937, y=1.1) -> (x*y=w935:dbl)
              }
            }
          }
        }
        "COD浓度（mg/L)" <- w866
      }
      frame "写入数据" {
        n560 = flat-sequence {
          tunnel: w952 -> [w963]
          tunnel: w951 -> [w962]
          tunnel: w948 -> [w956]
          tunnel: w947 -> [w955]
          tunnel: [w958] -> w946
          tunnel: [w957] -> w945
          tunnel: [w954] -> w944
          tunnel: [w953] -> w943
          tunnel: [w969] -> w949
          tunnel: [w970] -> w950
          tunnel: w946 -> [w970]
          tunnel: w945 -> [w969]
          tunnel: w944 -> [w968]
          tunnel: w943 -> [w967]
          frame #0 {
            n561 = Dequeue Element(queue=w962, error in (no error)=w955) -> (queue out=w954:refnum<queue>, element=w961:cluster{"starting address":u16, "values":u16[]}, error out=w953:errorcluster)  [unwired: 1 in, 1 out]
            n562 = Unbundle By Name(w961) -> ("starting address"=w960:u16, "values"=w959:u16[])
            n563 = call <vilib>:"Write Multiple Registers.vi"("error in (no error)"=w956, "values"=w959, "starting address"=w960, "MB session in"=w963) -> ("error out"=w957:errorcluster, "MB session out"=w958:refnum<class "MB_Master_Serial.lvclass">)  [unwired: 6 in]
          }
          frame #1 {
            n564 = Get Queue Status(queue=w968, error in (no error)=w967) -> (# elements in queue=w966:i32)  [unwired: 1 in, 7 out]
            n565 = Equal To 0?(x=w966) -> (x = 0?=w965:bool)
            n566 = case shown="假" w965 {
              tunnel: [enum16{"读取数据", "写入数据", "读取写入DATABASE", "读取参数"}."写入数据" ("枚举") enum16{"读取数据", "写入数据", "读取写入DATABASE", "读取参数"}."读取数据" ("枚举")] -> w964
              frame False {
              }
              frame True {
              }
            }
            n567 = local write "枚举"(w964) -> ()
          }
        }
      }
      frame "读取写入DATABASE" {
        w1008 = "CODMn" ("table")
        n568 = Dequeue Element(queue=w1039, timeout in ms (-1)=1000 ("超时毫秒(-1)"), error in (no error)=w1038) -> (element=w1046:T7)  [unwired: 3 out]
        n569 = Unbundle By Name(w1046) -> ("starting address"=w1045:u16, "number of holding registers"=w1044:u16)
        n570 = call <vilib>:"Read Holding Registers.vi"("error in (no error)"=w1040, "quantity"=w1044, "starting address"=w1045, "MB session in"=w1041) -> ("error out"=w1042:errorcluster, "Registers"=w1004:u16[], "MB session out"=w1043:refnum<class "MB_Master_Serial.lvclass">)  [unwired: 5 in]
        "DATABASE" <- w1004
        n571 = Split 1D Array(array=w1004, index=3 ("索引")) -> (first subarray=w1036:u16[], second subarray=w1025:u16[])
        n572 = global read "系统变量.vi" "运行模式"() -> (w988:enum16{"维护模式", "常规模式", "应急模式", "质控模式"})
        n573 = case shown="\"常规模式\"" w988 {
          tunnel: ["M" ("单位") "N" ("单位") "hd" ("单位") "hd" ("单位")] -> w987
          frame "维护模式", Default {
          }
          frame "常规模式" {
          }
          frame "应急模式" {
          }
          frame "质控模式" {
          }
        }
        n574 = Index Array(array=w1036) -> (element #1=w1034:u16, element #2=w1033:u16, element #3=w1032:u16)  [unwired: 3 in]
        n575 = Index Array(array=w1025) -> (element #1=w973:u16, element #2=w1029:u16, element #3=w1028:u16, element #4=w1027:u16, element #5=w1026:u16)  [unwired: 5 in]
        n576 = Index Array(array=w1025, index=6 ("索引")) -> (element=w1023:u16)
        n577 = To Single Precision Float(number=w973) -> (single precision float=w975:sgl)
        n578 = Divide(x=w975, y=sgl 100.0) -> (x/y=w974:sgl)
        n579 = Less Or Equal?(x=w974, y=sgl 0.01) -> (x <= y?=w979:bool)
        n580 = local read "标样浓度 2"() -> (w1002:dbl)
        n581 = case shown="真" w979 {
          tunnel: [w1069 w1070] -> w977
          tunnel: w974 -> [w1069 _]
          frame False {
          }
          frame True {
            n582 = Random Number (0-1)() -> (number: 0 to 1=w1073:dbl)
            n583 = Increment(x=w1073) -> (x+1=w1071:dbl)
            n584 = Divide(x=w1071, y=sgl 100.0) -> (x/y=w1070:dbl)
          }
        }
        n585 = Build Array(w1034, w1033, w1032) -> (w1031:u16[])
        n586 = To Single Precision Float(number=w1029) -> (single precision float=w993:sgl)
        n587 = To Single Precision Float(number=w1028) -> (single precision float=w994:sgl)
        n588 = To Single Precision Float(number=w1027) -> (single precision float=w995:sgl)
        n589 = To Single Precision Float(number=w1026) -> (single precision float=w1020:sgl)
        n590 = property on="基本量程" class="Enum (严格)"() -> ("Value"=w978:enum16{"10mL", "20mL"})  [unwired: 2 in, 2 out]
        n591 = case shown="\"10mL\", 默认" w978 {
          tunnel: w977 -> [w1049 w1059]
          tunnel: [w1047 w1058] -> w976
          frame "10mL", Default {
            n592 = Less Or Equal?(x=w1049, y=2.0) -> (x <= y?=w1052:bool)
            n593 = Greater?(x=w1049, y=0.0) -> (0:w1051:bool)
            n594 = And(x=w1052, y=w1051) -> (x .and. y?=w1048:bool)
            n595 = case shown="真" w1048 {
              tunnel: w1049 -> [w1054 w1057]
              tunnel: [w1054 w1055] -> w1047
              frame False {
              }
              frame True {
                n596 = Multiply(x=w1057, y=1.1) -> (x*y=w1055:dbl)
              }
            }
          }
          frame "20mL" {
            n597 = Less Or Equal?(x=w1059, y=4.0) -> (x <= y?=w1063:bool)
            n598 = Greater?(x=w1059, y=0.0) -> (0:w1062:bool)
            n599 = And(x=w1063, y=w1062) -> (x .and. y?=w1060:bool)
            n600 = case shown="真" w1060 {
              tunnel: w1059 -> [w1065 w1068]
              tunnel: [w1065 w1066] -> w1058
              frame False {
              }
              frame True {
                n601 = Multiply(x=w1068, y=1.1) -> (x*y=w1066:dbl)
              }
            }
          }
        }
        n602 = Divide(x=w1002, y=100.0) -> (x/y=w992:dbl)
        n603 = To Single Precision Float(number=w1023) -> (single precision float=w981:sgl)
        n604 = call "HexToDate.vi"("数组"=w1031) -> ("DATE"=w1035:timestamp[])  [unwired: 10 in]
        n605 = global read "COD测量模式全局.vi" "测量模式"() -> (w983:string)
        n606 = Divide(x=w1020, y=sgl 1000.0) -> (x/y=w996:sgl)
        n607 = Index Array(array=w1035) -> (element=w1030:timestamp)  [unwired: 1 in]
        n608 = Format Into String(format string="w%05d" ("格式字符串"), u32 1019 ("因子编码")) -> (resulting string=w991:string)  [unwired: 2 in, 1 out]
        n609 = local read "温度"() -> (w986:dbl)
        n610 = disable-structure shown="启用" {
          disable-tunnel: w985 -> [w1076 _]
          disable-tunnel: w976 -> [w1075 _]
          frame Disabled {
            n611 = Greater Or Equal?(x=w1075, y=sgl 10.0) -> (x >= y?=w1074:bool)
            n612 = case shown="假" w1074 {
              tunnel: w1076 -> [w1079 w1087]
              frame False {
                # "自动切换量程"
                n613 = local write "枚举"(enum16{"读取数据", "写入数据", "读取写入DATABASE", "读取参数"}."写入数据" ("枚举")) -> ()
                n614 = Bundle By Name(cluster=cluster{"starting address":u16, "values":u16[]} {"starting address"=0, "values"=[]}, "starting address"=u16 4276, "values"=u16[] [0]) -> (w1082:cluster{"starting address":u16, "values":u16[]})
                n615 = Enqueue Element(queue=w1079, element=w1082) -> ()  [unwired: 2 in, 3 out]
              }
              frame True {
                n616 = local write "枚举"(enum16{"读取数据", "写入数据", "读取写入DATABASE", "读取参数"}."写入数据" ("枚举")) -> ()
                n617 = Bundle By Name(cluster=cluster{"starting address":u16, "values":u16[]} {"starting address"=0, "values"=[]}, "starting address"=u16 4276, "values"=u16[] [1]) -> (w1088:cluster{"starting address":u16, "values":u16[]})
                n618 = Enqueue Element(queue=w1087, element=w1088) -> ()  [unwired: 2 in, 3 out]
              }
            }
          }
          frame Enabled {
          }
        }
        n619 = local read "当前选用的校准"() -> (w982:i32)
        n620 = Bundle(cluster=T6 {"时间"=timestamp(0 s since 1904-01-01), "测量模式"="", "数据类型"="", "检测值"=0.0, "单位"="", "数据标识"="", "因子编码"="", "标样参考值"=0.0, "ORP-A"=0.0, "ORP-B"=0.0, "ORP-K"=0.0, "COD滴定值"=0.0, "高锰酸钾滴定数"=0.0, "温度"=0.0} ("data"), "时间"=w1030, "测量模式"=w983, "数据类型"=w987, "检测值"=w976, "单位"="mg/L", "数据标识"="N", "因子编码"=w991, "标样参考值"=w992, "ORP-A"=w993, "ORP-B"=w994, "ORP-K"=w995, "COD滴定值"=w996, "高锰酸钾滴定数"=w981, "温度"=w986) -> (w984:T6)
        "data" <- w984
        n621 = Build Array("时间", "测量模式", "数据类型", "检测值", "单位", "数据标识", "因子编码", "标样参考值", "ORPA", "ORPB", "ORPK", "COD滴定值", "高锰酸钾滴定数", "温度") -> (w1007:string[])
        "columns" <- w1007
        n622 = global write "COD浓度全局变量.vi" "COD浓度（mg/L)"(w976) -> ()
        n623 = global write "COD读取DATA全局.vi" "data"(w984) -> ()
        n624 = case shown="6" w982 {
          tunnel: w981 -> [w1090 w1091 w1092 w1093 w1094 w1095]
          frame 1, Default {
            n625 = local write "泵滴定数1"(w1090) -> ()
          }
          frame 2 {
            n626 = local write "泵滴定数2"(w1091) -> ()
          }
          frame 3 {
            n627 = local write "泵滴定数3"(w1092) -> ()
          }
          frame 4 {
            n628 = local write "泵滴定数4"(w1093) -> ()
          }
          frame 5 {
            n629 = local write "泵滴定数5"(w1094) -> ()
          }
          frame 6 {
            n630 = local write "泵滴定数6"(w1095) -> ()
          }
        }
        n631 = call "数据写入database.vi"("data"=w984, "columns"=w1007, "table"=w1008) -> ()  [unwired: 9 in]
        "table 输入" <- w1008
      }
      frame "读取参数" {
        n632 = Dequeue Element(queue=w1106, timeout in ms (-1)=1000 ("超时毫秒(-1)"), error in (no error)=w1105) -> (element=w1112:T7)  [unwired: 3 out]
        n633 = local write "枚举"(enum16{"读取数据", "写入数据", "读取写入DATABASE", "读取参数"}."读取数据" ("枚举")) -> ()
        n634 = Unbundle By Name(w1112) -> ("starting address"=w1111:u16, "number of holding registers"=w1110:u16)
        n635 = local read "读取KB值"() -> (w1101:bool)
        n636 = call <vilib>:"Read Holding Registers.vi"("error in (no error)"=w1107, "quantity"=w1110, "starting address"=w1111, "MB session in"=w1108) -> ("error out"=w1100:errorcluster, "Registers"=w1104:u16[], "MB session out"=w1102:refnum<class "MB_Master_Serial.lvclass">)  [unwired: 5 in]
        "读取参数" <- w1104
        n637 = case shown="真" w1101 {
          tunnel: w1104 -> [w1122 w1144]
          tunnel: w1100 -> [_ w1146]
          frame False {
            n638 = Index Array(array=w1122) -> (element #1=w1116:u16, element #2=w1135:u16, element #3=w1134:u16, element #4=w1114:u16, element #5=w1133:u16, element #6=w1132:u16, element #7=w1131:u16, element #8=w1130:u16, element #9=w1129:u16, element #10=w1128:u16, element #11=w1127:u16, element #12=w1126:u16, element #13=w1125:u16, element #14=w1124:u16, element #15=w1123:u16, element #16=w1121:u16)  [unwired: 16 in]
            n639 = local write "浓度"(w1134) -> ()
            n640 = local write "水样"(w1132) -> ()
            n641 = local write "硫酸"(w1125) -> ()
            n642 = local write "标液"(w1130) -> ()
            n643 = Divide(x=w1116, y=u16 10) -> (x/y=w1117:dbl)
            n644 = local write "恒温时间"(w1135) -> ()
            n645 = local write "基本量程"(w1133) -> ()
            n646 = local write "加标回收"(w1128) -> ()
            n647 = local write "高锰酸钾"(w1127) -> ()
            n648 = local write "草酸钠"(w1126) -> ()
            n649 = local write "零点泵计量数 2"(w1124) -> ()
            n650 = local write "标度泵计量数 2"(w1123) -> ()
            n651 = local write "蒸馏水"(w1131) -> ()
            n652 = local write "质控样"(w1129) -> ()
            n653 = Divide(x=w1114, y=u16 100) -> (x/y=w1113:dbl)
            n654 = Divide(x=w1121, y=u16 100) -> (x/y=w1120:dbl)
            n655 = local write "温度"(w1117) -> ()
            n656 = local write "修正系数 2"(w1113) -> ()
            n657 = local write "浓度 2"(w1120) -> ()
          }
          frame True {
            n658 = case shown="错误" w1146 {
              tunnel: ["读取成功" ("消息") "读取失败" ("消息")] -> w1145
              frame No Error {
              }
              frame Error {
              }
            }
            n659 = call "浮点CDAB转换COD.vi"("数组"=w1144) -> ("数组 2"=w1143:sgl[])  [unwired: 10 in]
            n660 = Array To Cluster(array=w1143) -> (cluster=w1142:T14)
            n661 = One Button Dialog(message=w1145) -> ()  [unwired: 1 in, 1 out]
            n662 = Unbundle By Name(w1142) -> ("数组 2[0]"=w1141:sgl, "数组 2[1]"=w1140:sgl, "数组 2[2]"=w1138:sgl, "数组 2[3]"=w1137:sgl)
            n663 = Bundle By Name(cluster=T1 {"k"=0.0, "b"=0.0, "k 2"=0.0, "b 2"=0.0, "写入"=FALSE} ("读取方程系数"), "k"=w1141, "b"=w1140, "k 2"=w1138, "b 2"=w1137) -> (w1136:T1)
            n664 = local write "读取方程系数"(w1136) -> ()
          }
        }
      }
    }
    n665 = Unbundle By Name(w851) -> ("status"=w852:bool)
    n666 = Not(x=w852) -> (.not. x?=→"通讯状态":bool)
    "数值" <- w850
  }
  n667 = call-dynamic "Close Session.vi"("error in (no error)"=w18, "MB_Serial session"=w17) -> ()  [unwired: 9 in, 1 out]
